vi "Standard Normal distribution.vi"() -> ()   [LabVIEW 2023]
uses:
  <vilib>/numeric/Random Number (Range) U64.vi
  <vilib>/numeric/Random Number (Range) DBL.vi
  <vilib>/numeric/sub_Random U32.vi
  <vilib>/gmath/NI_Gmath.lvlib
panel:
  in  "stop":bool
  out "xyGraph":cluster{"X":dbl, "Y":dbl}[](graph)=[{"X"=-6.09, "Y"=3.526399235495381e-09}, {"X"=-6.08, "Y"=3.747643729676039e-09}, {"X"=-6.07, "Y"=3.982370733890178e-09}, {"X"=-6.06, "Y"=4.231376288039894e-09}, {"X"=-6.05, "Y"=4.4955018310132455e-09}, {"X"=-6.04, "Y"=4.775636692282276e-09}, {"X"=-6.03, "Y"=5.072720714470481e-09}, {"X"=-6.02, "Y"=5.38774701344276e-09}, {"X"=-6.01, "Y"=5.7217648827798965e-09}, {"X"=-6.0, "Y"=6.075882849823286e-09}, {"X"=-5.99, "Y"=6.451271890811751e-09}, {"X"=-5.98, "Y"=6.8491688129857586e-09}, {"X"=-5.97, "Y"=7.270879811900108e-09}, {"X"=-5.96, "Y"=7.717784212570529e-09}, {"X"=-5.95, "Y"=8.191338403479174e-09}, {"X"=-5.94, "Y"=8.693079972880173e-09}, {"X"=-5.93, "Y"=9.22463205728272e-09}, {"X"=-5.92, "Y"=9.78770791244118e-09}, {"X"=-5.91, "Y"=1.0384115717656327e-08}, {"X"=-5.9, "Y"=1.1015763624682308e-08}, {"X"=-5.89, "Y"=1.168466506304987e-08}, {"X"=-5.88, "Y"=1.239294431415013e-08}, {"X"=-5.87, "Y"=1.3142842366982143e-08}, {"X"=-5.86, "Y"=1.3936723069047392e-08}, {"X"=-5.85, "Y"=1.4777079586480055e-08}, {"X"=-5.84, "Y"=1.5666541188132572e-08}, {"X"=-5.83, "Y"=1.6607880368992047e-08}, {"X"=-5.82, "Y"=1.7604020328985783e-08}, {"X"=-5.81, "Y"=1.865804282394618e-08}, {"X"=-5.8, "Y"=1.9773196406244675e-08}, {"X"=-5.79, "Y"=2.0952905073377047e-08}, {"X"=-5.78, "Y"=2.2200777343579013e-08}, {"X"=-5.77, "Y"=2.352061577839084e-08}, {"X"=-5.76, "Y"=2.4916426972950992e-08}, {"X"=-5.75, "Y"=2.6392432035705735e-08}, {"X"=-5.74, "Y"=2.795307758015465e-08}, {"X"=-5.73, "Y"=2.960304725223005e-08}, {"X"=-5.72, "Y"=3.134727381791979e-08}, {"X"=-5.71, "Y"=3.319095183679538e-08}, {"X"=-5.7, "Y"=3.513955094820434e-08}, {"X"=-5.69, "Y"=3.7198829798016034e-08}, {"X"=-5.68, "Y"=3.9374850634998504e-08}, {"X"=-5.67, "Y"=4.167399460712351e-08}, {"X"=-5.66, "Y"=4.410297778937308e-08}, {"X"=-5.65, "Y"=4.666886797594257e-08}, {"X"=-5.64, "Y"=4.937910227110449e-08}, {"X"=-5.63, "Y"=5.2241505514424374e-08}, {"X"=-5.62, "Y"=5.526430957749716e-08}, {"X"=-5.61, "Y"=5.84561735709005e-08}, {"X"=-5.6, "Y"=6.182620500165857e-08}, {"X"=-5.59, "Y"=6.538398192315145e-08}, {"X"=-5.58, "Y"=6.913957612112398e-08}, {"X"=-5.57, "Y"=7.310357738120935e-08}, {"X"=-5.56, "Y"=7.728711888522921e-08}, {"X"=-5.55, "Y"=8.17019037854322e-08}, {"X"=-5.54, "Y"=8.636023300780988e-08}, {"X"=-5.53, "Y"=9.127503433766477e-08}, {"X"=-5.52, "Y"=9.645989284273384e-08}, {"X"=-5.51, "Y"=1.0192908269135293e-07}, {"X"=-5.5, "Y"=1.0769760042543276e-07}, {"X"=-5.49, "Y"=1.1378119975034591e-07}, {"X"=-5.48, "Y"=1.201964279062823e-07}, {"X"=-5.47, "Y"=1.2696066368812932e-07}, {"X"=-5.46, "Y"=1.3409215718354753e-07}, {"X"=-5.45, "Y"=1.4161007130161178e-07}, {"X"=-5.44, "Y"=1.495345251671592e-07}, {"X"=-5.43, "Y"=1.5788663945889064e-07}, {"X"=-5.42, "Y"=1.6668858377222828e-07}, {"X"=-5.41, "Y"=1.7596362609104592e-07}, {"X"=-5.4, "Y"=1.8573618445552897e-07}, {"X"=-5.39, "Y"=1.9603188091675758e-07}, {"X"=-5.38, "Y"=2.0687759787196552e-07}, {"X"=-5.37, "Y"=2.1830153687797888e-07}, {"X"=-5.36, "Y"=2.3033328004392066e-07}, {"X"=-5.35, "Y"=2.4300385410805355e-07}, {"X"=-5.34, "Y"=2.5634579730745934e-07}, {"X"=-5.33, "Y"=2.7039322915329305e-07}, {"X"=-5.32, "Y"=2.851819232283976e-07}, {"X"=-5.31, "Y"=3.007493831283838e-07}, {"X"=-5.3, "Y"=3.171349216715976e-07}, {"X"=-5.29, "Y"=3.3437974350798003e-07}, {"X"=-5.28, "Y"=3.525270312614038e-07}, {"X"=-5.27, "Y"=3.7162203534495063e-07}, {"X"=-5.26, "Y"=3.9171216759348166e-07}, {"X"=-5.25, "Y"=4.1284709886299984e-07}, {"X"=-5.24, "Y"=4.350788607515109e-07}, {"X"=-5.23, "Y"=4.584619516015329e-07}, {"X"=-5.22, "Y"=4.830534469499683e-07}, {"X"=-5.21, "Y"=5.08913114596766e-07}, {"X"=-5.2, "Y"=5.361035344697615e-07}, {"X"=-5.19, "Y"=5.64690223469076e-07}, {"X"=-5.18, "Y"=5.947417654807764e-07}, {"X"=-5.17, "Y"=6.263299467558902e-07}, {"X"=-5.16, "Y"=6.595298968575217e-07}, {"X"=-5.15, "Y"=6.944202353855339e-07}, {"X"=-5.14, "Y"=7.310832246953503e-07}, {"X"=-5.13, "Y"=7.696049288345129e-07}, {"X"=-5.12, "Y"=8.100753789281346e-07}, {"X"=-5.11, "Y"=8.52588745251786e-07}, {"X"=-5.1, "Y"=8.972435162383337e-07}, {"X"=-5.09, "Y"=9.441426846730874e-07}, {"X"=-5.08, "Y"=9.93393941339912e-07}, {"X"=-5.07, "Y"=1.0451098763893177e-06}, {"X"=-5.06, "Y"=1.0994081887082052e-06}, {"X"=-5.05, "Y"=1.1564119035797834e-06}, {"X"=-5.04, "Y"=1.216249598931318e-06}, {"X"=-5.03, "Y"=1.2790556404765742e-06}, {"X"=-5.02, "Y"=1.3449704260694445e-06}, {"X"=-5.01, "Y"=1.4141406395950037e-06}, {"X"=-5.0, "Y"=1.4867195147342979e-06}, {"X"=-4.99, "Y"=1.5628671089492902e-06}, {"X"=-4.98, "Y"=1.6427505880450713e-06}, {"X"=-4.97, "Y"=1.7265445216770736e-06}, {"X"=-4.96, "Y"=1.8144311901820306e-06}, {"X"=-4.95, "Y"=1.906600903122811e-06}, {"X"=-4.94, "Y"=2.0032523299484894e-06}, {"X"=-4.93, "Y"=2.10459284318313e-06}, {"X"=-4.92, "Y"=2.2108388745684212e-06}, {"X"=-4.91, "Y"=2.322216284597997e-06}, {"X"=-4.9, "Y"=2.438960745893352e-06}, {"X"=-4.89, "Y"=2.5613181408845447e-06}, {"X"=-4.88, "Y"=2.6895449742715237e-06}, {"X"=-4.87, "Y"=2.823908800755821e-06}, {"X"=-4.86, "Y"=2.964688668545273e-06}, {"X"=-4.85, "Y"=3.112175579148945e-06}, {"X"=-4.84, "Y"=3.266672963993275e-06}, {"X"=-4.83, "Y"=3.428497178405039e-06}, {"X"=-4.82, "Y"=3.5979780135212474e-06}, {"X"=-4.81, "Y"=3.775459226701349e-06}, {"X"=-4.8, "Y"=3.961299091032075e-06}, {"X"=-4.79, "Y"=4.155870964531201e-06}, {"X"=-4.78, "Y"=4.359563879671637e-06}, {"X"=-4.77, "Y"=4.5727831538641446e-06}, {"X"=-4.76, "Y"=4.795951021552522e-06}, {"X"=-4.75, "Y"=5.029507288592446e-06}, {"X"=-4.74, "Y"=5.273910009601304e-06}, {"X"=-4.73, "Y"=5.529636188984052e-06}, {"X"=-4.72, "Y"=5.797182506357288e-06}, {"X"=-4.71, "Y"=6.077066067111116e-06}, {"X"=-4.7, "Y"=6.36982517886709e-06}, {"X"=-4.69, "Y"=6.676020154607462e-06}, {"X"=-4.68, "Y"=6.996234143270405e-06}, {"X"=-4.67, "Y"=7.331073988623946e-06}, {"X"=-4.66, "Y"=7.681171117250455e-06}, {"X"=-4.65, "Y"=8.047182456492295e-06}, {"X"=-4.64, "Y"=8.429791383228772e-06}, {"X"=-4.63, "Y"=8.829708704374098e-06}, {"X"=-4.62, "Y"=9.247673670005617e-06}, {"X"=-4.61, "Y"=9.684455020051437e-06}, {"X"=-4.6, "Y"=1.014085206548676e-05}, {"X"=-4.59, "Y"=1.0617695805008393e-05}, {"X"=-4.58, "Y"=1.111585007817779e-05}, {"X"=-4.57, "Y"=1.1636212756042669e-05}, {"X"=-4.56, "Y"=1.21797169702687e-05}, {"X"=-4.55, "Y"=1.2747332381833467e-05}, {"X"=-4.54, "Y"=1.334006649035584e-05}, {"X"=-4.53, "Y"=1.3958965985154772e-05}, {"X"=-4.52, "Y"=1.4605118139152942e-05}, {"X"=-4.51, "Y"=1.527965224676162e-05}, {"X"=-4.5, "Y"=1.5983741106905478e-05}, {"X"=-4.49, "Y"=1.671860255236507e-05}, {"X"=-4.48, "Y"=1.748550102663914e-05}, {"X"=-4.47, "Y"=1.828574920954738e-05}, {"X"=-4.46, "Y"=1.9120709692817737e-05}, {"X"=-4.45, "Y"=1.999179670692279e-05}, {"X"=-4.44, "Y"=2.0900477900450407e-05}, {"X"=-4.43, "Y"=2.184827617331647e-05}, {"X"=-4.42, "Y"=2.283677156514692e-05}, {"X"=-4.41, "Y"=2.38676032001796e-05}, {"X"=-4.4, "Y"=2.4942471290053535e-05}, {"X"=-4.39, "Y"=2.6063139195878346e-05}, {"X"=-4.38, "Y"=2.723143555099261e-05}, {"X"=-4.37, "Y"=2.8449256445844308e-05}, {"X"=-4.36, "Y"=2.97185676764422e-05}, {"X"=-4.35, "Y"=3.1041407057850266e-05}, {"X"=-4.34, "Y"=3.241988680421378e-05}, {"X"=-4.33, "Y"=3.385619597682789e-05}, {"X"=-4.32, "Y"=3.5352603001773097e-05}, {"X"=-4.31, "Y"=3.69114582586662e-05}, {"X"=-4.3, "Y"=3.853519674208713e-05}, {"X"=-4.29, "Y"=4.022634079726497e-05}, {"X"=-4.28, "Y"=4.198750293161732e-05}, {"X"=-4.27, "Y"=4.382138870375812e-05}, {"X"=-4.26, "Y"=4.5730799691601314e-05}, {"X"=-4.25, "Y"=4.771863654120495e-05}, {"X"=-4.24, "Y"=4.978790209801209e-05}, {"X"=-4.23, "Y"=5.1941704622159776e-05}, {"X"=-4.22, "Y"=5.4183261089540144e-05}, {"X"=-4.21, "Y"=5.651590058030741e-05}, {"X"=-4.2, "Y"=5.8943067756539855e-05}, {"X"=-4.19, "Y"=6.146832643076922e-05}, {"X"=-4.18, "Y"=6.40953632271061e-05}, {"X"=-4.17, "Y"=6.682799133669061e-05}, {"X"=-4.16, "Y"=6.967015436921434e-05}, {"X"=-4.15, "Y"=7.262593030225234e-05}, {"X"=-4.14, "Y"=7.569953553016121e-05}, {"X"=-4.13, "Y"=7.889532901429309e-05}, {"X"=-4.12, "Y"=8.2217816536286e-05}, {"X"=-4.11, "Y"=8.567165505618186e-05}, {"X"=-4.1, "Y"=8.926165717713293e-05}, {"X"=-4.09, "Y"=9.299279571844591e-05}, {"X"=-4.08, "Y"=9.687020839871927e-05}, {"X"=-4.07, "Y"=0.00010089920263081443}, {"X"=-4.06, "Y"=0.00010508526043040049}, {"X"=-4.05, "Y"=0.00010943404343980055}, {"X"=-4.04, "Y"=0.00011395139806886461}, {"X"=-4.03, "Y"=0.00011864336075456578}, {"X"=-4.02, "Y"=0.00012351616334102368}, {"X"=-4.01, "Y"=0.00012857623858162108}, {"X"=-4.0, "Y"=0.00013383022576488537}, {"X"=-3.99, "Y"=0.00013928497646575994}, {"X"=-3.98, "Y"=0.00014494756042389106}, {"X"=-3.97, "Y"=0.0001508252715505178}, {"X"=-3.96, "Y"=0.00015692563406553226}, {"X"=-3.95, "Y"=0.00016325640876624202}, {"X"=-3.94, "Y"=0.00016982559942934359}, {"X"=-3.93, "Y"=0.00017664145934757092}, {"X"=-3.92, "Y"=0.0001837124980024571}, {"X"=-3.91, "Y"=0.00019104748787459762}, {"X"=-3.9, "Y"=0.00019865547139277272}, {"X"=-3.89, "Y"=0.00020654576802322548}, {"X"=-3.88, "Y"=0.00021472798150036704}, {"X"=-3.87, "Y"=0.0002232120072001021}, {"X"=-3.86, "Y"=0.00023200803965694238}, {"X"=-3.85, "Y"=0.00024112658022599324}, {"X"=-3.84, "Y"=0.00025057844489086075}, {"X"=-3.83, "Y"=0.00026037477221844247}, {"X"=-3.82, "Y"=0.000270527031461521}, {"X"=-3.81, "Y"=0.0002810470308099863}, {"X"=-3.8, "Y"=0.00029194692579146027}, {"X"=-3.79, "Y"=0.0003032392278220042}, {"X"=-3.78, "Y"=0.0003149368129075219}, {"X"=-3.77, "Y"=0.00032705293049637503}, {"X"=-3.76, "Y"=0.0003396012124836548}, {"X"=-3.75, "Y"=0.00035259568236744546}, {"X"=-3.74, "Y"=0.000366050764557335}, {"X"=-3.73, "Y"=0.00037998129383532146}, {"X"=-3.72, "Y"=0.0003944025249691562}, {"X"=-3.71, "Y"=0.0004093301424780789}, {"X"=-3.7, "Y"=0.00042478027055075143}, {"X"=-3.69, "Y"=0.0004407694831151325}, {"X"=-3.68, "Y"=0.00045731481405985675}, {"X"=-3.67, "Y"=0.00047443376760662064}, {"X"=-3.66, "Y"=0.0004921443288328931}, {"X"=-3.65, "Y"=0.0005104649743441856}, {"X"=-3.64, "Y"=0.0005294146830949348}, {"X"=-3.63, "Y"=0.0005490129473569587}, {"X"=-3.62, "Y"=0.0005692797838342526}, {"X"=-3.61, "Y"=0.0005902357449227856}, {"X"=-3.6, "Y"=0.0006119019301137719}, {"X"=-3.59, "Y"=0.0006342999975387576}, {"X"=-3.58, "Y"=0.0006574521756546766}, {"X"=-3.57, "Y"=0.0006813812750668921}, {"X"=-3.56, "Y"=0.0007061107004880362}, {"X"=-3.55, "Y"=0.0007316644628303109}, {"X"=-3.54, "Y"=0.0007580671914287103}, {"X"=-3.53, "Y"=0.00078534414639247}, {"X"=-3.52, "Y"=0.0008135212310818085}, {"X"=-3.51, "Y"=0.0008426250047069028}, {"X"=-3.5, "Y"=0.0008726826950457602}, {"X"=-3.49, "Y"=0.0009037222112775245}, {"X"=-3.48, "Y"=0.0009357721569274798}, {"X"=-3.47, "Y"=0.0009688618429198459}, {"X"=-3.46, "Y"=0.0010030213007342376}, {"X"=-3.45, "Y"=0.0010382812956614103}, {"X"=-3.44, "Y"=0.0010746733401537356}, {"X"=-3.43, "Y"=0.0011122297072655649}, {"X"=-3.42, "Y"=0.0011509834441784845}, {"X"=-3.41, "Y"=0.0011909683858061168}, {"X"=-3.4, "Y"=0.00123221916847302}, {"X"=-3.39, "Y"=0.001274771243661833}, {"X"=-3.38, "Y"=0.0013186608918227423}, {"X"=-3.37, "Y"=0.0013639252362389036}, {"X"=-3.36, "Y"=0.001410602256941385}, {"X"=-3.35, "Y"=0.0014587308046667459}, {"X"=-3.34, "Y"=0.0015083506148503075}, {"X"=-3.33, "Y"=0.0015595023216476915}, {"X"=-3.32, "Y"=0.0016122274719771244}, {"X"=-3.31, "Y"=0.0016665685395745797}, {"X"=-3.3, "Y"=0.0017225689390536812}, {"X"=-3.29, "Y"=0.0017802730399618788}, {"X"=-3.28, "Y"=0.0018397261808242812}, {"X"=-3.27, "Y"=0.0019009746831660803}, {"X"=-3.26, "Y"=0.001964065865504376}, {"X"=-3.25, "Y"=0.002029048057299768}, {"X"=-3.24, "Y"=0.002095970612857942}, {"X"=-3.23, "Y"=0.0021648839251710624}, {"X"=-3.22, "Y"=0.0022358394396885385}, {"X"=-3.21, "Y"=0.0023088896680064958}, {"X"=-3.2, "Y"=0.0023840882014648404}, {"X"=-3.19, "Y"=0.0024614897246407006}, {"X"=-3.18, "Y"=0.002541150028726522}, {"X"=-3.17, "Y"=0.0026231260247810244}, {"X"=-3.16, "Y"=0.0027074757568407003}, {"X"=-3.15, "Y"=0.002794258414879447}, {"X"=-3.14, "Y"=0.002883534347603439}, {"X"=-3.13, "Y"=0.002975365075068254}, {"X"=-3.12, "Y"=0.0030698133011047403}, {"X"=-3.11, "Y"=0.0031669429255400815}, {"X"=-3.1, "Y"=0.0032668190561999186}, {"X"=-3.09, "Y"=0.0033695080206774812}, {"X"=-3.08, "Y"=0.003475077377854938}, {"X"=-3.07, "Y"=0.0035835959291623614}, {"X"=-3.06, "Y"=0.003695133729559035}, {"X"=-3.05, "Y"=0.0038097620982218104}, {"X"=-3.04, "Y"=0.003927553628924779}, {"X"=-3.03, "Y"=0.00404858220009443}, {"X"=-3.02, "Y"=0.004172922984523962}, {"X"=-3.01, "Y"=0.00430065245873045}, {"X"=-3.0, "Y"=0.0044318484119380075}, {"X"=-2.99, "Y"=0.004566589954670145}, {"X"=-2.98, "Y"=0.004704957526933979}, {"X"=-2.97, "Y"=0.004847032905978945}, {"X"=-2.96, "Y"=0.004992899213612376}, {"X"=-2.95, "Y"=0.005142640923053939}, {"X"=-2.94, "Y"=0.00529634386531102}, {"X"=-2.93, "Y"=0.005454095235056545}, {"X"=-2.92, "Y"=0.005615983595990969}, {"X"=-2.91, "Y"=0.005782098885669473}, {"X"=-2.9, "Y"=0.005952532419775854}, {"X"=-2.89, "Y"=0.006127376895823688}, {"X"=-2.88, "Y"=0.0063067263962659275}, {"X"=-2.87, "Y"=0.006490676390993364}, {"X"=-2.86, "Y"=0.00667932373920262}, {"X"=-2.85, "Y"=0.006872766690613971}, {"X"=-2.84, "Y"=0.007071104886019449}, {"X"=-2.83, "Y"=0.007274439357141218}, {"X"=-2.82, "Y"=0.007482872525780564}, {"X"=-2.81, "Y"=0.007696508202237322}, {"X"=-2.8, "Y"=0.007915451582979969}, {"X"=-2.79, "Y"=0.008139809247546021}, {"X"=-2.78, "Y"=0.008369689154653033}, {"X"=-2.77, "Y"=0.008605200637499673}, {"X"=-2.76, "Y"=0.008846454398237232}, {"X"=-2.75, "Y"=0.009093562501591053}, {"X"=-2.74, "Y"=0.009346638367612283}, {"X"=-2.73, "Y"=0.009605796763539587}, {"X"=-2.72, "Y"=0.009871153794751132}, {"X"=-2.71, "Y"=0.010142826894787078}, {"X"=-2.7, "Y"=0.010420934814422592}, {"X"=-2.69, "Y"=0.010705597609772188}, {"X"=-2.68, "Y"=0.010996936629405572}, {"X"=-2.67, "Y"=0.011295074500456135}, {"X"=-2.66, "Y"=0.011600135113702562}, {"X"=-2.65, "Y"=0.01191224360760518}, {"X"=-2.64, "Y"=0.012231526351277971}, {"X"=-2.63, "Y"=0.012558110926378211}, {"X"=-2.62, "Y"=0.012892126107895304}, {"X"=-2.61, "Y"=0.013233701843821374}, {"X"=-2.6, "Y"=0.013582969233685615}, {"X"=-2.59, "Y"=0.013940060505935825}, {"X"=-2.58, "Y"=0.014305108994149692}, {"X"=-2.57, "Y"=0.014678249112060044}, {"X"=-2.56, "Y"=0.01505961632737745}, {"X"=-2.55, "Y"=0.015449347134395174}, {"X"=-2.54, "Y"=0.015847579025360818}, {"X"=-2.53, "Y"=0.016254450460600506}, {"X"=-2.52, "Y"=0.016670100837381057}, {"X"=-2.51, "Y"=0.017094670457496956}, {"X"=-2.5, "Y"=0.01752830049356854}, {"X"=-2.49, "Y"=0.017971132954039633}, {"X"=-2.48, "Y"=0.01842331064686205}, {"X"=-2.47, "Y"=0.018884977141856163}, {"X"=-2.46, "Y"=0.019356276731736965}, {"X"=-2.45, "Y"=0.019837354391795313}, {"X"=-2.44, "Y"=0.02032835573822584}, {"X"=-2.43, "Y"=0.020829426985092186}, {"X"=-2.42, "Y"=0.021340714899922786}, {"X"=-2.41, "Y"=0.021862366757929387}, {"X"=-2.4, "Y"=0.0223945302948429}, {"X"=-2.39, "Y"=0.022937353658360693}, {"X"=-2.38, "Y"=0.023490985358201367}, {"X"=-2.37, "Y"=0.02405557421476297}, {"X"=-2.36, "Y"=0.024631269306382507}, {"X"=-2.35, "Y"=0.025218219915194382}, {"X"=-2.34, "Y"=0.02581657547158769}, {"X"=-2.33, "Y"=0.026426485497261724}, {"X"=-2.32, "Y"=0.027048099546881785}, {"X"=-2.31, "Y"=0.027681567148336573}, {"X"=-2.3, "Y"=0.02832703774160119}, {"X"=-2.29, "Y"=0.028984660616209416}, {"X"=-2.28, "Y"=0.029654584847341278}, {"X"=-2.27, "Y"=0.03033695923053164}, {"X"=-2.26, "Y"=0.031031932215008273}, {"X"=-2.25, "Y"=0.03173965183566742}, {"X"=-2.24, "Y"=0.032460265643697445}, {"X"=-2.23, "Y"=0.03319392063586112}, {"X"=-2.22, "Y"=0.033940763182449186}, {"X"=-2.21, "Y"=0.03470093895391882}, {"X"=-2.2, "Y"=0.035474592846231424}, {"X"=-2.19, "Y"=0.03626186890490622}, {"X"=-2.18, "Y"=0.037062910247806474}, {"X"=-2.17, "Y"=0.03787785898667748}, {"X"=-2.16, "Y"=0.03870685614745561}, {"X"=-2.15, "Y"=0.03955004158937022}, {"X"=-2.14, "Y"=0.04040755392286031}, {"X"=-2.13, "Y"=0.041279530426330424}, {"X"=-2.12, "Y"=0.04216610696177031}, {"X"=-2.11, "Y"=0.04306741788926574}, {"X"=-2.1, "Y"=0.0439835959804272}, {"X"=-2.09, "Y"=0.0449147723307671}, {"X"=-2.08, "Y"=0.045861076271054894}, {"X"=-2.07, "Y"=0.04682263527768316}, {"X"=-2.06, "Y"=0.047799574882077034}, {"X"=-2.05, "Y"=0.04879201857918277}, {"X"=-2.04, "Y"=0.049800087735070775}, {"X"=-2.03, "Y"=0.05082390149369121}, {"X"=-2.02, "Y"=0.051863576682820565}, {"X"=-2.01, "Y"=0.05291922771924032}, {"X"=-2.0, "Y"=0.05399096651318806}, {"X"=-1.99, "Y"=0.05507890237212577}, {"X"=-1.98, "Y"=0.05618314190386805}, {"X"=-1.97, "Y"=0.05730378891911713}, {"X"=-1.96, "Y"=0.058440944333451476}, {"X"=-1.95, "Y"=0.059594706068816075}, {"X"=-1.94, "Y"=0.06076516895456478}, {"X"=-1.93, "Y"=0.061952424628105164}, {"X"=-1.92, "Y"=0.06315656143519865}, {"X"=-1.91, "Y"=0.06437766432996936}, {"X"=-1.9, "Y"=0.0656158147746766}, {"X"=-1.89, "Y"=0.06687109063930716}, {"X"=-1.88, "Y"=0.06814356610104459}, {"X"=-1.87, "Y"=0.06943331154367419}, {"X"=-1.86, "Y"=0.07074039345698338}, {"X"=-1.85, "Y"=0.072064874336218}, {"X"=-1.84, "Y"=0.07340681258165689}, {"X"=-1.83, "Y"=0.0747662623983676}, {"X"=-1.82, "Y"=0.07614327369620731}, {"X"=-1.81, "Y"=0.07753789199013399}, {"X"=-1.8, "Y"=0.07895015830089415}, {"X"=-1.79, "Y"=0.08038010905615417}, {"X"=-1.78, "Y"=0.08182777599214282}, {"X"=-1.77, "Y"=0.08329318605587446}, {"X"=-1.76, "Y"=0.08477636130802224}, {"X"=-1.75, "Y"=0.08627731882651153}, {"X"=-1.74, "Y"=0.08779607061090564}, {"X"=-1.73, "Y"=0.089332623487655}, {"X"=-1.72, "Y"=0.09088697901628288}, {"X"=-1.71, "Y"=0.09245913339658068}, {"X"=-1.7, "Y"=0.09404907737688695}, {"X"=-1.69, "Y"=0.09565679616352402}, {"X"=-1.68, "Y"=0.09728226933146752}, {"X"=-1.67, "Y"=0.09892547073632373}, {"X"=-1.66, "Y"=0.10058636842769057}, {"X"=-1.65, "Y"=0.10226492456397804}, {"X"=-1.64, "Y"=0.10396109532876424}, {"X"=-1.63, "Y"=0.10567483084876363}, {"X"=-1.62, "Y"=0.1074060751134838}, {"X"=-1.61, "Y"=0.10915476589664735}, {"X"=-1.6, "Y"=0.11092083467945554}, {"X"=-1.59, "Y"=0.11270420657577056}, {"X"=-1.58, "Y"=0.11450480025929236}, {"X"=-1.57, "Y"=0.1163225278928071}, {"X"=-1.56, "Y"=0.11815729505958228}, {"X"=-1.55, "Y"=0.12000900069698558}, {"X"=-1.54, "Y"=0.12187753703240178}, {"X"=-1.53, "Y"=0.12376278952152314}, {"X"=-1.52, "Y"=0.12566463678908815}, {"X"=-1.51, "Y"=0.12758295057214186}, {"X"=-1.5, "Y"=0.12951759566589174}, {"X"=-1.49, "Y"=0.13146842987223106}, {"X"=-1.48, "Y"=0.13343530395100234}, {"X"=-1.47, "Y"=0.1354180615740713}, {"X"=-1.46, "Y"=0.13741653928228179}, {"X"=-1.45, "Y"=0.13943056644536028}, {"X"=-1.44, "Y"=0.1414599652248388}, {"X"=-1.43, "Y"=0.14350455054006242}, {"X"=-1.42, "Y"=0.1455641300373476}, {"X"=-1.41, "Y"=0.14763850406235574}, {"X"=-1.4, "Y"=0.14972746563574488}, {"X"=-1.39, "Y"=0.1518308004321617}, {"X"=-1.38, "Y"=0.15394828676263372}, {"X"=-1.37, "Y"=0.15607969556042084}, {"X"=-1.36, "Y"=0.15822479037038303}, {"X"=-1.35, "Y"=0.1603833273419196}, {"X"=-1.34, "Y"=0.16255505522553412}, {"X"=-1.33, "Y"=0.1647397153730768}, {"X"=-1.32, "Y"=0.1669370417417138}, {"X"=-1.31, "Y"=0.1691467609016724}, {"X"=-1.3, "Y"=0.17136859204780736}, {"X"=-1.29, "Y"=0.173602247015033}, {"X"=-1.28, "Y"=0.17584743029766237}, {"X"=-1.27, "Y"=0.1781038390726936}, {"X"=-1.26, "Y"=0.18037116322708033}, {"X"=-1.25, "Y"=0.18264908538902191}, {"X"=-1.24, "Y"=0.1849372809633053}, {"X"=-1.23, "Y"=0.18723541817072956}, {"X"=-1.22, "Y"=0.18954315809164027}, {"X"=-1.21, "Y"=0.1918601547135994}, {"X"=-1.2, "Y"=0.19418605498321298}, {"X"=-1.19, "Y"=0.19652049886213654}, {"X"=-1.18, "Y"=0.1988631193872759}, {"X"=-1.17, "Y"=0.2012135427351974}, {"X"=-1.16, "Y"=0.20357138829075944}, {"X"=-1.15, "Y"=0.20593626871997478}, {"X"=-1.14, "Y"=0.20830779004710837}, {"X"=-1.13, "Y"=0.21068555173601533}, {"X"=-1.12, "Y"=0.21306914677571784}, {"X"=-1.11, "Y"=0.2154581617702197}, {"X"=-1.1, "Y"=0.21785217703255055}, {"X"=-1.09, "Y"=0.22025076668303326}, {"X"=-1.08, "Y"=0.22265349875176116}, {"X"=-1.07, "Y"=0.22505993528526969}, {"X"=-1.06, "Y"=0.2274696324573859}, {"X"=-1.05, "Y"=0.22988214068423302}, {"X"=-1.04, "Y"=0.2322970047433662}, {"X"=-1.03, "Y"=0.23471376389701185}, {"X"=-1.02, "Y"=0.23713195201937962}, {"X"=-1.01, "Y"=0.23955109772801336}, {"X"=-1.0, "Y"=0.24197072451914337}, {"X"=-0.99, "Y"=0.2443903509069996}, {"X"=-0.98, "Y"=0.24680949056704274}, {"X"=-0.97, "Y"=0.24922765248306594}, {"X"=-0.96, "Y"=0.2516443410981171}, {"X"=-0.95, "Y"=0.254059056469189}, {"X"=-0.94, "Y"=0.25647129442562033}, {"X"=-0.93, "Y"=0.25888054673114885}, {"X"=-0.92, "Y"=0.26128630124955315}, {"X"=-0.91, "Y"=0.2636880421138182}, {"X"=-0.9, "Y"=0.2660852498987548}, {"X"=-0.89, "Y"=0.2684774017970024}, {"X"=-0.88, "Y"=0.27086397179833804}, {"X"=-0.87, "Y"=0.2732444308722162}, {"X"=-0.86, "Y"=0.27561824715345673}, {"X"=-0.85, "Y"=0.2779848861309965}, {"X"=-0.84, "Y"=0.2803438108396206}, {"X"=-0.83, "Y"=0.28269448205458025}, {"X"=-0.82, "Y"=0.28503635848900727}, {"X"=-0.81, "Y"=0.2873688969940283}, {"X"=-0.8, "Y"=0.28969155276148273}, {"X"=-0.79, "Y"=0.2920037795291414}, {"X"=-0.78, "Y"=0.2943050297883251}, {"X"=-0.77, "Y"=0.2965947549938157}, {"X"=-0.76, "Y"=0.29887240577595275}, {"X"=-0.75, "Y"=0.30113743215480443}, {"X"=-0.74, "Y"=0.30338928375630014}, {"X"=-0.73, "Y"=0.30562741003020993}, {"X"=-0.72, "Y"=0.30785126046985295}, {"X"=-0.71, "Y"=0.31006028483341613}, {"X"=-0.7, "Y"=0.31225393336676127}, {"X"=-0.69, "Y"=0.31443165702759734}, {"X"=-0.68, "Y"=0.31659290771089277}, {"X"=-0.67, "Y"=0.3187371384754015}, {"X"=-0.66, "Y"=0.3208638037711725}, {"X"=-0.65, "Y"=0.3229723596679143}, {"X"=-0.64, "Y"=0.3250622640840822}, {"X"=-0.63, "Y"=0.3271329770165545}, {"X"=-0.62, "Y"=0.3291839607707648}, {"X"=-0.61, "Y"=0.33121468019115297}, {"X"=-0.6, "Y"=0.33322460289179967}, {"X"=-0.59, "Y"=0.33521319948710615}, {"X"=-0.58, "Y"=0.3371799438223806}, {"X"=-0.57, "Y"=0.33912431320419223}, {"X"=-0.56, "Y"=0.34104578863035256}, {"X"=-0.55, "Y"=0.3429438550193839}, {"X"=-0.54, "Y"=0.3448180014393334}, {"X"=-0.53, "Y"=0.34666772133579166}, {"X"=-0.52, "Y"=0.3484925127589745}, {"X"=-0.51, "Y"=0.3502918785897258}, {"X"=-0.5, "Y"=0.3520653267642995}, {"X"=-0.49, "Y"=0.3538123704977797}, {"X"=-0.48, "Y"=0.3555325285059971}, {"X"=-0.47, "Y"=0.35722532522580086}, {"X"=-0.46, "Y"=0.35889029103354464}, {"X"=-0.45, "Y"=0.36052696246164795}, {"X"=-0.44, "Y"=0.3621348824130922}, {"X"=-0.43, "Y"=0.3637136003737134}, {"X"=-0.42, "Y"=0.3652626726221539}, {"X"=-0.41, "Y"=0.3667816624373361}, {"X"=-0.4, "Y"=0.36827014030332333}, {"X"=-0.39, "Y"=0.36972768411143236}, {"X"=-0.38, "Y"=0.37115387935946603}, {"X"=-0.37, "Y"=0.3725483193479334}, {"X"=-0.36, "Y"=0.3739106053731284}, {"X"=-0.35, "Y"=0.3752403469169379}, {"X"=-0.34, "Y"=0.376537161833254}, {"X"=-0.33, "Y"=0.37780067653086463}, {"X"=-0.32, "Y"=0.3790305261527017}, {"X"=-0.31, "Y"=0.38022635475132494}, {"X"=-0.3, "Y"=0.38138781546052414}, {"X"=-0.29, "Y"=0.38251457066292405}, {"X"=-0.28, "Y"=0.3836062921534786}, {"X"=-0.27, "Y"=0.3846626612987428}, {"X"=-0.26, "Y"=0.3856833691918161}, {"X"=-0.25, "Y"=0.3866681168028493}, {"X"=-0.24, "Y"=0.38761661512501416}, {"X"=-0.23, "Y"=0.3885285853158359}, {"X"=-0.22, "Y"=0.38940375883379047}, {"X"=-0.21, "Y"=0.39024187757007434}, {"X"=-0.2, "Y"=0.3910426939754559}, {"X"=-0.19, "Y"=0.3918059711821211}, {"X"=-0.18, "Y"=0.3925314831204289}, {"X"=-0.17, "Y"=0.3932190146304972}, {"X"=-0.16, "Y"=0.3938683615685408}, {"X"=-0.15, "Y"=0.39447933090788895}, {"X"=-0.14, "Y"=0.39505174083461125}, {"X"=-0.13, "Y"=0.3955854208376874}, {"X"=-0.12, "Y"=0.3960802117936561}, {"X"=-0.11, "Y"=0.3965359660456858}, {"X"=-0.1, "Y"=0.3969525474770118}, {"X"=-0.09, "Y"=0.39732983157868834}, {"X"=-0.08, "Y"=0.3976677055116089}, {"X"=-0.07, "Y"=0.39796606816275104}, {"X"=-0.06, "Y"=0.39822483019560695}, {"X"=-0.05, "Y"=0.39844391409476404}, {"X"=-0.04, "Y"=0.39862325420460504}, {"X"=-0.03, "Y"=0.39876279676209975}, {"X"=-0.02, "Y"=0.3988624999236661}, {"X"=-0.01, "Y"=0.39892233378608216}, {"X"=0.0, "Y"=0.3989422804014327}, {"X"=-0.0, "Y"=0.3989422804014327}, {"X"=0.01, "Y"=0.39892233378608216}, {"X"=0.02, "Y"=0.3988624999236661}, {"X"=0.03, "Y"=0.39876279676209975}, {"X"=0.04, "Y"=0.39862325420460504}, {"X"=0.05, "Y"=0.39844391409476404}, {"X"=0.06, "Y"=0.39822483019560695}, {"X"=0.07, "Y"=0.39796606816275104}, {"X"=0.08, "Y"=0.3976677055116089}, {"X"=0.09, "Y"=0.39732983157868834}, {"X"=0.1, "Y"=0.3969525474770118}, {"X"=0.11, "Y"=0.3965359660456858}, {"X"=0.12, "Y"=0.3960802117936561}, {"X"=0.13, "Y"=0.3955854208376874}, {"X"=0.14, "Y"=0.39505174083461125}, {"X"=0.15, "Y"=0.39447933090788895}, {"X"=0.16, "Y"=0.3938683615685408}, {"X"=0.17, "Y"=0.3932190146304972}, {"X"=0.18, "Y"=0.3925314831204289}, {"X"=0.19, "Y"=0.3918059711821211}, {"X"=0.2, "Y"=0.3910426939754559}, {"X"=0.21, "Y"=0.39024187757007434}, {"X"=0.22, "Y"=0.38940375883379047}, {"X"=0.23, "Y"=0.3885285853158359}, {"X"=0.24, "Y"=0.38761661512501416}, {"X"=0.25, "Y"=0.3866681168028493}, {"X"=0.26, "Y"=0.3856833691918161}, {"X"=0.27, "Y"=0.3846626612987428}, {"X"=0.28, "Y"=0.3836062921534786}, {"X"=0.29, "Y"=0.38251457066292405}, {"X"=0.3, "Y"=0.38138781546052414}, {"X"=0.31, "Y"=0.38022635475132494}, {"X"=0.32, "Y"=0.3790305261527017}, {"X"=0.33, "Y"=0.37780067653086463}, {"X"=0.34, "Y"=0.376537161833254}, {"X"=0.35, "Y"=0.3752403469169379}, {"X"=0.36, "Y"=0.3739106053731284}, {"X"=0.37, "Y"=0.3725483193479334}, {"X"=0.38, "Y"=0.37115387935946603}, {"X"=0.39, "Y"=0.36972768411143236}, {"X"=0.4, "Y"=0.36827014030332333}, {"X"=0.41, "Y"=0.3667816624373361}, {"X"=0.42, "Y"=0.3652626726221539}, {"X"=0.43, "Y"=0.3637136003737134}, {"X"=0.44, "Y"=0.3621348824130922}, {"X"=0.45, "Y"=0.36052696246164795}, {"X"=0.46, "Y"=0.35889029103354464}, {"X"=0.47, "Y"=0.35722532522580086}, {"X"=0.48, "Y"=0.3555325285059971}, {"X"=0.49, "Y"=0.3538123704977797}, {"X"=0.5, "Y"=0.3520653267642995}, {"X"=0.51, "Y"=0.3502918785897258}, {"X"=0.52, "Y"=0.3484925127589745}, {"X"=0.53, "Y"=0.34666772133579166}, {"X"=0.54, "Y"=0.3448180014393334}, {"X"=0.55, "Y"=0.3429438550193839}, {"X"=0.56, "Y"=0.34104578863035256}, {"X"=0.57, "Y"=0.33912431320419223}, {"X"=0.58, "Y"=0.3371799438223806}, {"X"=0.59, "Y"=0.33521319948710615}, {"X"=0.6, "Y"=0.33322460289179967}, {"X"=0.61, "Y"=0.33121468019115297}, {"X"=0.62, "Y"=0.3291839607707648}, {"X"=0.63, "Y"=0.3271329770165545}, {"X"=0.64, "Y"=0.3250622640840822}, {"X"=0.65, "Y"=0.3229723596679143}, {"X"=0.66, "Y"=0.3208638037711725}, {"X"=0.67, "Y"=0.3187371384754015}, {"X"=0.68, "Y"=0.31659290771089277}, {"X"=0.69, "Y"=0.31443165702759734}, {"X"=0.7, "Y"=0.31225393336676127}, {"X"=0.71, "Y"=0.31006028483341613}, {"X"=0.72, "Y"=0.30785126046985295}, {"X"=0.73, "Y"=0.30562741003020993}, {"X"=0.74, "Y"=0.30338928375630014}, {"X"=0.75, "Y"=0.30113743215480443}, {"X"=0.76, "Y"=0.29887240577595275}, {"X"=0.77, "Y"=0.2965947549938157}, {"X"=0.78, "Y"=0.2943050297883251}, {"X"=0.79, "Y"=0.2920037795291414}, {"X"=0.8, "Y"=0.28969155276148273}, {"X"=0.81, "Y"=0.2873688969940283}, {"X"=0.82, "Y"=0.28503635848900727}, {"X"=0.83, "Y"=0.28269448205458025}, {"X"=0.84, "Y"=0.2803438108396206}, {"X"=0.85, "Y"=0.2779848861309965}, {"X"=0.86, "Y"=0.27561824715345673}, {"X"=0.87, "Y"=0.2732444308722162}, {"X"=0.88, "Y"=0.27086397179833804}, {"X"=0.89, "Y"=0.2684774017970024}, {"X"=0.9, "Y"=0.2660852498987548}, {"X"=0.91, "Y"=0.2636880421138182}, {"X"=0.92, "Y"=0.26128630124955315}, {"X"=0.93, "Y"=0.25888054673114885}, {"X"=0.94, "Y"=0.25647129442562033}, {"X"=0.95, "Y"=0.254059056469189}, {"X"=0.96, "Y"=0.2516443410981171}, {"X"=0.97, "Y"=0.24922765248306594}, {"X"=0.98, "Y"=0.24680949056704274}, {"X"=0.99, "Y"=0.2443903509069996}, {"X"=1.0, "Y"=0.24197072451914337}, {"X"=1.01, "Y"=0.23955109772801336}, {"X"=1.02, "Y"=0.23713195201937962}, {"X"=1.03, "Y"=0.23471376389701185}, {"X"=1.04, "Y"=0.2322970047433662}, {"X"=1.05, "Y"=0.22988214068423302}, {"X"=1.06, "Y"=0.2274696324573859}, {"X"=1.07, "Y"=0.22505993528526969}, {"X"=1.08, "Y"=0.22265349875176116}, {"X"=1.09, "Y"=0.22025076668303326}, {"X"=1.1, "Y"=0.21785217703255055}, {"X"=1.11, "Y"=0.2154581617702197}, {"X"=1.12, "Y"=0.21306914677571784}, {"X"=1.13, "Y"=0.21068555173601533}, {"X"=1.14, "Y"=0.20830779004710837}, {"X"=1.15, "Y"=0.20593626871997478}, {"X"=1.16, "Y"=0.20357138829075944}, {"X"=1.17, "Y"=0.2012135427351974}, {"X"=1.18, "Y"=0.1988631193872759}, {"X"=1.19, "Y"=0.19652049886213654}, {"X"=1.2, "Y"=0.19418605498321298}, {"X"=1.21, "Y"=0.1918601547135994}, {"X"=1.22, "Y"=0.18954315809164027}, {"X"=1.23, "Y"=0.18723541817072956}, {"X"=1.24, "Y"=0.1849372809633053}, {"X"=1.25, "Y"=0.18264908538902191}, {"X"=1.26, "Y"=0.18037116322708033}, {"X"=1.27, "Y"=0.1781038390726936}, {"X"=1.28, "Y"=0.17584743029766237}, {"X"=1.29, "Y"=0.173602247015033}, {"X"=1.3, "Y"=0.17136859204780736}, {"X"=1.31, "Y"=0.1691467609016724}, {"X"=1.32, "Y"=0.1669370417417138}, {"X"=1.33, "Y"=0.1647397153730768}, {"X"=1.34, "Y"=0.16255505522553412}, {"X"=1.35, "Y"=0.1603833273419196}, {"X"=1.36, "Y"=0.15822479037038303}, {"X"=1.37, "Y"=0.15607969556042084}, {"X"=1.38, "Y"=0.15394828676263372}, {"X"=1.39, "Y"=0.1518308004321617}, {"X"=1.4, "Y"=0.14972746563574488}, {"X"=1.41, "Y"=0.14763850406235574}, {"X"=1.42, "Y"=0.1455641300373476}, {"X"=1.43, "Y"=0.14350455054006242}, {"X"=1.44, "Y"=0.1414599652248388}, {"X"=1.45, "Y"=0.13943056644536028}, {"X"=1.46, "Y"=0.13741653928228179}, {"X"=1.47, "Y"=0.1354180615740713}, {"X"=1.48, "Y"=0.13343530395100234}, {"X"=1.49, "Y"=0.13146842987223106}, {"X"=1.5, "Y"=0.12951759566589174}, {"X"=1.51, "Y"=0.12758295057214186}, {"X"=1.52, "Y"=0.12566463678908815}, {"X"=1.53, "Y"=0.12376278952152314}, {"X"=1.54, "Y"=0.12187753703240178}, {"X"=1.55, "Y"=0.12000900069698558}, {"X"=1.56, "Y"=0.11815729505958228}, {"X"=1.57, "Y"=0.1163225278928071}, {"X"=1.58, "Y"=0.11450480025929236}, {"X"=1.59, "Y"=0.11270420657577056}, {"X"=1.6, "Y"=0.11092083467945554}, {"X"=1.61, "Y"=0.10915476589664735}, {"X"=1.62, "Y"=0.1074060751134838}, {"X"=1.63, "Y"=0.10567483084876363}, {"X"=1.64, "Y"=0.10396109532876424}, {"X"=1.65, "Y"=0.10226492456397804}, {"X"=1.66, "Y"=0.10058636842769057}, {"X"=1.67, "Y"=0.09892547073632373}, {"X"=1.68, "Y"=0.09728226933146752}, {"X"=1.69, "Y"=0.09565679616352402}, {"X"=1.7, "Y"=0.09404907737688695}, {"X"=1.71, "Y"=0.09245913339658068}, {"X"=1.72, "Y"=0.09088697901628288}, {"X"=1.73, "Y"=0.089332623487655}, {"X"=1.74, "Y"=0.08779607061090564}, {"X"=1.75, "Y"=0.08627731882651153}, {"X"=1.76, "Y"=0.08477636130802224}, {"X"=1.77, "Y"=0.08329318605587446}, {"X"=1.78, "Y"=0.08182777599214282}, {"X"=1.79, "Y"=0.08038010905615417}, {"X"=1.8, "Y"=0.07895015830089415}, {"X"=1.81, "Y"=0.07753789199013399}, {"X"=1.82, "Y"=0.07614327369620731}, {"X"=1.83, "Y"=0.0747662623983676}, {"X"=1.84, "Y"=0.07340681258165689}, {"X"=1.85, "Y"=0.072064874336218}, {"X"=1.86, "Y"=0.07074039345698338}, {"X"=1.87, "Y"=0.06943331154367419}, {"X"=1.88, "Y"=0.06814356610104459}, {"X"=1.89, "Y"=0.06687109063930716}, {"X"=1.9, "Y"=0.0656158147746766}, {"X"=1.91, "Y"=0.06437766432996936}, {"X"=1.92, "Y"=0.06315656143519865}, {"X"=1.93, "Y"=0.061952424628105164}, {"X"=1.94, "Y"=0.06076516895456478}, {"X"=1.95, "Y"=0.059594706068816075}, {"X"=1.96, "Y"=0.058440944333451476}, {"X"=1.97, "Y"=0.05730378891911713}, {"X"=1.98, "Y"=0.05618314190386805}, {"X"=1.99, "Y"=0.05507890237212577}, {"X"=2.0, "Y"=0.05399096651318806}, {"X"=2.01, "Y"=0.05291922771924032}, {"X"=2.02, "Y"=0.051863576682820565}, {"X"=2.03, "Y"=0.05082390149369121}, {"X"=2.04, "Y"=0.049800087735070775}, {"X"=2.05, "Y"=0.04879201857918277}, {"X"=2.06, "Y"=0.047799574882077034}, {"X"=2.07, "Y"=0.04682263527768316}, {"X"=2.08, "Y"=0.045861076271054894}, {"X"=2.09, "Y"=0.0449147723307671}, {"X"=2.1, "Y"=0.0439835959804272}, {"X"=2.11, "Y"=0.04306741788926574}, {"X"=2.12, "Y"=0.04216610696177031}, {"X"=2.13, "Y"=0.041279530426330424}, {"X"=2.14, "Y"=0.04040755392286031}, {"X"=2.15, "Y"=0.03955004158937022}, {"X"=2.16, "Y"=0.03870685614745561}, {"X"=2.17, "Y"=0.03787785898667748}, {"X"=2.18, "Y"=0.037062910247806474}, {"X"=2.19, "Y"=0.03626186890490622}, {"X"=2.2, "Y"=0.035474592846231424}, {"X"=2.21, "Y"=0.03470093895391882}, {"X"=2.22, "Y"=0.033940763182449186}, {"X"=2.23, "Y"=0.03319392063586112}, {"X"=2.24, "Y"=0.032460265643697445}, {"X"=2.25, "Y"=0.03173965183566742}, {"X"=2.26, "Y"=0.031031932215008273}, {"X"=2.27, "Y"=0.03033695923053164}, {"X"=2.28, "Y"=0.029654584847341278}, {"X"=2.29, "Y"=0.028984660616209416}, {"X"=2.3, "Y"=0.02832703774160119}, {"X"=2.31, "Y"=0.027681567148336573}, {"X"=2.32, "Y"=0.027048099546881785}, {"X"=2.33, "Y"=0.026426485497261724}, {"X"=2.34, "Y"=0.02581657547158769}, {"X"=2.35, "Y"=0.025218219915194382}, {"X"=2.36, "Y"=0.024631269306382507}, {"X"=2.37, "Y"=0.02405557421476297}, {"X"=2.38, "Y"=0.023490985358201367}, {"X"=2.39, "Y"=0.022937353658360693}, {"X"=2.4, "Y"=0.0223945302948429}, {"X"=2.41, "Y"=0.021862366757929387}, {"X"=2.42, "Y"=0.021340714899922786}, {"X"=2.43, "Y"=0.020829426985092186}, {"X"=2.44, "Y"=0.02032835573822584}, {"X"=2.45, "Y"=0.019837354391795313}, {"X"=2.46, "Y"=0.019356276731736965}, {"X"=2.47, "Y"=0.018884977141856163}, {"X"=2.48, "Y"=0.01842331064686205}, {"X"=2.49, "Y"=0.017971132954039633}, {"X"=2.5, "Y"=0.01752830049356854}, {"X"=2.51, "Y"=0.017094670457496956}, {"X"=2.52, "Y"=0.016670100837381057}, {"X"=2.53, "Y"=0.016254450460600506}, {"X"=2.54, "Y"=0.015847579025360818}, {"X"=2.55, "Y"=0.015449347134395174}, {"X"=2.56, "Y"=0.01505961632737745}, {"X"=2.57, "Y"=0.014678249112060044}, {"X"=2.58, "Y"=0.014305108994149692}, {"X"=2.59, "Y"=0.013940060505935825}, {"X"=2.6, "Y"=0.013582969233685615}, {"X"=2.61, "Y"=0.013233701843821374}, {"X"=2.62, "Y"=0.012892126107895304}, {"X"=2.63, "Y"=0.012558110926378211}, {"X"=2.64, "Y"=0.012231526351277971}, {"X"=2.65, "Y"=0.01191224360760518}, {"X"=2.66, "Y"=0.011600135113702562}, {"X"=2.67, "Y"=0.011295074500456135}, {"X"=2.68, "Y"=0.010996936629405572}, {"X"=2.69, "Y"=0.010705597609772188}, {"X"=2.7, "Y"=0.010420934814422592}, {"X"=2.71, "Y"=0.010142826894787078}, {"X"=2.72, "Y"=0.009871153794751132}, {"X"=2.73, "Y"=0.009605796763539587}, {"X"=2.74, "Y"=0.009346638367612283}, {"X"=2.75, "Y"=0.009093562501591053}, {"X"=2.76, "Y"=0.008846454398237232}, {"X"=2.77, "Y"=0.008605200637499673}, {"X"=2.78, "Y"=0.008369689154653033}, {"X"=2.79, "Y"=0.008139809247546021}, {"X"=2.8, "Y"=0.007915451582979969}, {"X"=2.81, "Y"=0.007696508202237322}, {"X"=2.82, "Y"=0.007482872525780564}, {"X"=2.83, "Y"=0.007274439357141218}, {"X"=2.84, "Y"=0.007071104886019449}, {"X"=2.85, "Y"=0.006872766690613971}, {"X"=2.86, "Y"=0.00667932373920262}, {"X"=2.87, "Y"=0.006490676390993364}, {"X"=2.88, "Y"=0.0063067263962659275}, {"X"=2.89, "Y"=0.006127376895823688}, {"X"=2.9, "Y"=0.005952532419775854}, {"X"=2.91, "Y"=0.005782098885669473}, {"X"=2.92, "Y"=0.005615983595990969}, {"X"=2.93, "Y"=0.005454095235056545}, {"X"=2.94, "Y"=0.00529634386531102}, {"X"=2.95, "Y"=0.005142640923053939}, {"X"=2.96, "Y"=0.004992899213612376}, {"X"=2.97, "Y"=0.004847032905978945}, {"X"=2.98, "Y"=0.004704957526933979}, {"X"=2.99, "Y"=0.004566589954670145}, {"X"=3.0, "Y"=0.0044318484119380075}, {"X"=3.01, "Y"=0.00430065245873045}, {"X"=3.02, "Y"=0.004172922984523962}, {"X"=3.03, "Y"=0.00404858220009443}, {"X"=3.04, "Y"=0.003927553628924779}, {"X"=3.05, "Y"=0.0038097620982218104}, {"X"=3.06, "Y"=0.003695133729559035}, {"X"=3.07, "Y"=0.0035835959291623614}, {"X"=3.08, "Y"=0.003475077377854938}, {"X"=3.09, "Y"=0.0033695080206774812}, {"X"=3.1, "Y"=0.0032668190561999186}, {"X"=3.11, "Y"=0.0031669429255400815}, {"X"=3.12, "Y"=0.0030698133011047403}, {"X"=3.13, "Y"=0.002975365075068254}, {"X"=3.14, "Y"=0.002883534347603439}, {"X"=3.15, "Y"=0.002794258414879447}, {"X"=3.16, "Y"=0.0027074757568407003}, {"X"=3.17, "Y"=0.0026231260247810244}, {"X"=3.18, "Y"=0.002541150028726522}, {"X"=3.19, "Y"=0.0024614897246407006}, {"X"=3.2, "Y"=0.0023840882014648404}, {"X"=3.21, "Y"=0.0023088896680064958}, {"X"=3.22, "Y"=0.0022358394396885385}, {"X"=3.23, "Y"=0.0021648839251710624}, {"X"=3.24, "Y"=0.002095970612857942}, {"X"=3.25, "Y"=0.002029048057299768}, {"X"=3.26, "Y"=0.001964065865504376}, {"X"=3.27, "Y"=0.0019009746831660803}, {"X"=3.28, "Y"=0.0018397261808242812}, {"X"=3.29, "Y"=0.0017802730399618788}, {"X"=3.3, "Y"=0.0017225689390536812}, {"X"=3.31, "Y"=0.0016665685395745797}, {"X"=3.32, "Y"=0.0016122274719771244}, {"X"=3.33, "Y"=0.0015595023216476915}, {"X"=3.34, "Y"=0.0015083506148503075}, {"X"=3.35, "Y"=0.0014587308046667459}, {"X"=3.36, "Y"=0.001410602256941385}, {"X"=3.37, "Y"=0.0013639252362389036}, {"X"=3.38, "Y"=0.0013186608918227423}, {"X"=3.39, "Y"=0.001274771243661833}, {"X"=3.4, "Y"=0.00123221916847302}, {"X"=3.41, "Y"=0.0011909683858061168}, {"X"=3.42, "Y"=0.0011509834441784845}, {"X"=3.43, "Y"=0.0011122297072655649}, {"X"=3.44, "Y"=0.0010746733401537356}, {"X"=3.45, "Y"=0.0010382812956614103}, {"X"=3.46, "Y"=0.0010030213007342376}, {"X"=3.47, "Y"=0.0009688618429198459}, {"X"=3.48, "Y"=0.0009357721569274798}, {"X"=3.49, "Y"=0.0009037222112775245}, {"X"=3.5, "Y"=0.0008726826950457602}, {"X"=3.51, "Y"=0.0008426250047069028}, {"X"=3.52, "Y"=0.0008135212310818085}, {"X"=3.53, "Y"=0.00078534414639247}, {"X"=3.54, "Y"=0.0007580671914287103}, {"X"=3.55, "Y"=0.0007316644628303109}, {"X"=3.56, "Y"=0.0007061107004880362}, {"X"=3.57, "Y"=0.0006813812750668921}, {"X"=3.58, "Y"=0.0006574521756546766}, {"X"=3.59, "Y"=0.0006342999975387576}, {"X"=3.6, "Y"=0.0006119019301137719}, {"X"=3.61, "Y"=0.0005902357449227856}, {"X"=3.62, "Y"=0.0005692797838342526}, {"X"=3.63, "Y"=0.0005490129473569587}, {"X"=3.64, "Y"=0.0005294146830949348}, {"X"=3.65, "Y"=0.0005104649743441856}, {"X"=3.66, "Y"=0.0004921443288328931}, {"X"=3.67, "Y"=0.00047443376760662064}, {"X"=3.68, "Y"=0.00045731481405985675}, {"X"=3.69, "Y"=0.0004407694831151325}, {"X"=3.7, "Y"=0.00042478027055075143}, {"X"=3.71, "Y"=0.0004093301424780789}, {"X"=3.72, "Y"=0.0003944025249691562}, {"X"=3.73, "Y"=0.00037998129383532146}, {"X"=3.74, "Y"=0.000366050764557335}, {"X"=3.75, "Y"=0.00035259568236744546}, {"X"=3.76, "Y"=0.0003396012124836548}, {"X"=3.77, "Y"=0.00032705293049637503}, {"X"=3.78, "Y"=0.0003149368129075219}, {"X"=3.79, "Y"=0.0003032392278220042}, {"X"=3.8, "Y"=0.00029194692579146027}, {"X"=3.81, "Y"=0.0002810470308099863}, {"X"=3.82, "Y"=0.000270527031461521}, {"X"=3.83, "Y"=0.00026037477221844247}, {"X"=3.84, "Y"=0.00025057844489086075}, {"X"=3.85, "Y"=0.00024112658022599324}, {"X"=3.86, "Y"=0.00023200803965694238}, {"X"=3.87, "Y"=0.0002232120072001021}, {"X"=3.88, "Y"=0.00021472798150036704}, {"X"=3.89, "Y"=0.00020654576802322548}, {"X"=3.9, "Y"=0.00019865547139277272}, {"X"=3.91, "Y"=0.00019104748787459762}, {"X"=3.92, "Y"=0.0001837124980024571}, {"X"=3.93, "Y"=0.00017664145934757092}, {"X"=3.94, "Y"=0.00016982559942934359}, {"X"=3.95, "Y"=0.00016325640876624202}, {"X"=3.96, "Y"=0.00015692563406553226}, {"X"=3.97, "Y"=0.0001508252715505178}, {"X"=3.98, "Y"=0.00014494756042389106}, {"X"=3.99, "Y"=0.00013928497646575994}, {"X"=4.0, "Y"=0.00013383022576488537}, {"X"=4.01, "Y"=0.00012857623858162108}, {"X"=4.02, "Y"=0.00012351616334102368}, {"X"=4.03, "Y"=0.00011864336075456578}, {"X"=4.04, "Y"=0.00011395139806886461}, {"X"=4.05, "Y"=0.00010943404343980055}, {"X"=4.06, "Y"=0.00010508526043040049}, {"X"=4.07, "Y"=0.00010089920263081443}, {"X"=4.08, "Y"=9.687020839871927e-05}, {"X"=4.09, "Y"=9.299279571844591e-05}, {"X"=4.1, "Y"=8.926165717713293e-05}, {"X"=4.11, "Y"=8.567165505618186e-05}, {"X"=4.12, "Y"=8.2217816536286e-05}, {"X"=4.13, "Y"=7.889532901429309e-05}, {"X"=4.14, "Y"=7.569953553016121e-05}, {"X"=4.15, "Y"=7.262593030225234e-05}, {"X"=4.16, "Y"=6.967015436921434e-05}, {"X"=4.17, "Y"=6.682799133669061e-05}, {"X"=4.18, "Y"=6.40953632271061e-05}, {"X"=4.19, "Y"=6.146832643076922e-05}, {"X"=4.2, "Y"=5.8943067756539855e-05}, {"X"=4.21, "Y"=5.651590058030741e-05}, {"X"=4.22, "Y"=5.4183261089540144e-05}, {"X"=4.23, "Y"=5.1941704622159776e-05}, {"X"=4.24, "Y"=4.978790209801209e-05}, {"X"=4.25, "Y"=4.771863654120495e-05}, {"X"=4.26, "Y"=4.5730799691601314e-05}, {"X"=4.27, "Y"=4.382138870375812e-05}, {"X"=4.28, "Y"=4.198750293161732e-05}, {"X"=4.29, "Y"=4.022634079726497e-05}, {"X"=4.3, "Y"=3.853519674208713e-05}, {"X"=4.31, "Y"=3.69114582586662e-05}, {"X"=4.32, "Y"=3.5352603001773097e-05}, {"X"=4.33, "Y"=3.385619597682789e-05}, {"X"=4.34, "Y"=3.241988680421378e-05}, {"X"=4.35, "Y"=3.1041407057850266e-05}, {"X"=4.36, "Y"=2.97185676764422e-05}, {"X"=4.37, "Y"=2.8449256445844308e-05}, {"X"=4.38, "Y"=2.723143555099261e-05}, {"X"=4.39, "Y"=2.6063139195878346e-05}, {"X"=4.4, "Y"=2.4942471290053535e-05}, {"X"=4.41, "Y"=2.38676032001796e-05}, {"X"=4.42, "Y"=2.283677156514692e-05}, {"X"=4.43, "Y"=2.184827617331647e-05}, {"X"=4.44, "Y"=2.0900477900450407e-05}, {"X"=4.45, "Y"=1.999179670692279e-05}, {"X"=4.46, "Y"=1.9120709692817737e-05}, {"X"=4.47, "Y"=1.828574920954738e-05}, {"X"=4.48, "Y"=1.748550102663914e-05}, {"X"=4.49, "Y"=1.671860255236507e-05}, {"X"=4.5, "Y"=1.5983741106905478e-05}, {"X"=4.51, "Y"=1.527965224676162e-05}, {"X"=4.52, "Y"=1.4605118139152942e-05}, {"X"=4.53, "Y"=1.3958965985154772e-05}, {"X"=4.54, "Y"=1.334006649035584e-05}, {"X"=4.55, "Y"=1.2747332381833467e-05}, {"X"=4.56, "Y"=1.21797169702687e-05}, {"X"=4.57, "Y"=1.1636212756042669e-05}, {"X"=4.58, "Y"=1.111585007817779e-05}, {"X"=4.59, "Y"=1.0617695805008393e-05}, {"X"=4.6, "Y"=1.014085206548676e-05}, {"X"=4.61, "Y"=9.684455020051437e-06}, {"X"=4.62, "Y"=9.247673670005617e-06}, {"X"=4.63, "Y"=8.829708704374098e-06}, {"X"=4.64, "Y"=8.429791383228772e-06}, {"X"=4.65, "Y"=8.047182456492295e-06}, {"X"=4.66, "Y"=7.681171117250455e-06}, {"X"=4.67, "Y"=7.331073988623946e-06}, {"X"=4.68, "Y"=6.996234143270405e-06}, {"X"=4.69, "Y"=6.676020154607462e-06}, {"X"=4.7, "Y"=6.36982517886709e-06}, {"X"=4.71, "Y"=6.077066067111116e-06}, {"X"=4.72, "Y"=5.797182506357288e-06}, {"X"=4.73, "Y"=5.529636188984052e-06}, {"X"=4.74, "Y"=5.273910009601304e-06}, {"X"=4.75, "Y"=5.029507288592446e-06}, {"X"=4.76, "Y"=4.795951021552522e-06}, {"X"=4.77, "Y"=4.5727831538641446e-06}, {"X"=4.78, "Y"=4.359563879671637e-06}, {"X"=4.79, "Y"=4.155870964531201e-06}, {"X"=4.8, "Y"=3.961299091032075e-06}, {"X"=4.81, "Y"=3.775459226701349e-06}, {"X"=4.82, "Y"=3.5979780135212474e-06}, {"X"=4.83, "Y"=3.428497178405039e-06}, {"X"=4.84, "Y"=3.266672963993275e-06}, {"X"=4.85, "Y"=3.112175579148945e-06}, {"X"=4.86, "Y"=2.964688668545273e-06}, {"X"=4.87, "Y"=2.823908800755821e-06}, {"X"=4.88, "Y"=2.6895449742715237e-06}, {"X"=4.89, "Y"=2.5613181408845447e-06}, {"X"=4.9, "Y"=2.438960745893352e-06}, {"X"=4.91, "Y"=2.322216284597997e-06}, {"X"=4.92, "Y"=2.2108388745684212e-06}, {"X"=4.93, "Y"=2.10459284318313e-06}, {"X"=4.94, "Y"=2.0032523299484894e-06}, {"X"=4.95, "Y"=1.906600903122811e-06}, {"X"=4.96, "Y"=1.8144311901820306e-06}, {"X"=4.97, "Y"=1.7265445216770736e-06}, {"X"=4.98, "Y"=1.6427505880450713e-06}, {"X"=4.99, "Y"=1.5628671089492902e-06}, {"X"=5.0, "Y"=1.4867195147342979e-06}, {"X"=5.01, "Y"=1.4141406395950037e-06}, {"X"=5.02, "Y"=1.3449704260694445e-06}, {"X"=5.03, "Y"=1.2790556404765742e-06}, {"X"=5.04, "Y"=1.216249598931318e-06}, {"X"=5.05, "Y"=1.1564119035797834e-06}, {"X"=5.06, "Y"=1.0994081887082052e-06}, {"X"=5.07, "Y"=1.0451098763893177e-06}, {"X"=5.08, "Y"=9.93393941339912e-07}, {"X"=5.09, "Y"=9.441426846730874e-07}, {"X"=5.1, "Y"=8.972435162383337e-07}, {"X"=5.11, "Y"=8.52588745251786e-07}, {"X"=5.12, "Y"=8.100753789281346e-07}, {"X"=5.13, "Y"=7.696049288345129e-07}, {"X"=5.14, "Y"=7.310832246953503e-07}, {"X"=5.15, "Y"=6.944202353855339e-07}, {"X"=5.16, "Y"=6.595298968575217e-07}, {"X"=5.17, "Y"=6.263299467558902e-07}, {"X"=5.18, "Y"=5.947417654807764e-07}, {"X"=5.19, "Y"=5.64690223469076e-07}, {"X"=5.2, "Y"=5.361035344697615e-07}, {"X"=5.21, "Y"=5.08913114596766e-07}, {"X"=5.22, "Y"=4.830534469499683e-07}, {"X"=5.23, "Y"=4.584619516015329e-07}, {"X"=5.24, "Y"=4.350788607515109e-07}, {"X"=5.25, "Y"=4.1284709886299984e-07}, {"X"=5.26, "Y"=3.9171216759348166e-07}, {"X"=5.27, "Y"=3.7162203534495063e-07}, {"X"=5.28, "Y"=3.525270312614038e-07}, {"X"=5.29, "Y"=3.3437974350798003e-07}, {"X"=5.3, "Y"=3.171349216715976e-07}, {"X"=5.31, "Y"=3.007493831283838e-07}, {"X"=5.32, "Y"=2.851819232283976e-07}, {"X"=5.33, "Y"=2.7039322915329305e-07}, {"X"=5.34, "Y"=2.5634579730745934e-07}, {"X"=5.35, "Y"=2.4300385410805355e-07}, {"X"=5.36, "Y"=2.3033328004392066e-07}, {"X"=5.37, "Y"=2.1830153687797888e-07}, {"X"=5.38, "Y"=2.0687759787196552e-07}, {"X"=5.39, "Y"=1.9603188091675758e-07}, {"X"=5.4, "Y"=1.8573618445552897e-07}, {"X"=5.41, "Y"=1.7596362609104592e-07}, {"X"=5.42, "Y"=1.6668858377222828e-07}, {"X"=5.43, "Y"=1.5788663945889064e-07}, {"X"=5.44, "Y"=1.495345251671592e-07}, {"X"=5.45, "Y"=1.4161007130161178e-07}, {"X"=5.46, "Y"=1.3409215718354753e-07}, {"X"=5.47, "Y"=1.2696066368812932e-07}, {"X"=5.48, "Y"=1.201964279062823e-07}, {"X"=5.49, "Y"=1.1378119975034591e-07}, {"X"=5.5, "Y"=1.0769760042543276e-07}, {"X"=5.51, "Y"=1.0192908269135293e-07}, {"X"=5.52, "Y"=9.645989284273384e-08}, {"X"=5.53, "Y"=9.127503433766477e-08}, {"X"=5.54, "Y"=8.636023300780988e-08}, {"X"=5.55, "Y"=8.17019037854322e-08}, {"X"=5.56, "Y"=7.728711888522921e-08}, {"X"=5.57, "Y"=7.310357738120935e-08}, {"X"=5.58, "Y"=6.913957612112398e-08}, {"X"=5.59, "Y"=6.538398192315145e-08}, {"X"=5.6, "Y"=6.182620500165857e-08}, {"X"=5.61, "Y"=5.84561735709005e-08}, {"X"=5.62, "Y"=5.526430957749716e-08}, {"X"=5.63, "Y"=5.2241505514424374e-08}, {"X"=5.64, "Y"=4.937910227110449e-08}, {"X"=5.65, "Y"=4.666886797594257e-08}, {"X"=5.66, "Y"=4.410297778937308e-08}, {"X"=5.67, "Y"=4.167399460712351e-08}, {"X"=5.68, "Y"=3.9374850634998504e-08}, {"X"=5.69, "Y"=3.7198829798016034e-08}, {"X"=5.7, "Y"=3.513955094820434e-08}, {"X"=5.71, "Y"=3.319095183679538e-08}, {"X"=5.72, "Y"=3.134727381791979e-08}, {"X"=5.73, "Y"=2.960304725223005e-08}, {"X"=5.74, "Y"=2.795307758015465e-08}, {"X"=5.75, "Y"=2.6392432035705735e-08}, {"X"=5.76, "Y"=2.4916426972950992e-08}, {"X"=5.77, "Y"=2.352061577839084e-08}, {"X"=5.78, "Y"=2.2200777343579013e-08}, {"X"=5.79, "Y"=2.0952905073377047e-08}, {"X"=5.8, "Y"=1.9773196406244675e-08}, {"X"=5.81, "Y"=1.865804282394618e-08}, {"X"=5.82, "Y"=1.7604020328985783e-08}, {"X"=5.83, "Y"=1.6607880368992047e-08}, {"X"=5.84, "Y"=1.5666541188132572e-08}, {"X"=5.85, "Y"=1.4777079586480055e-08}, {"X"=5.86, "Y"=1.3936723069047392e-08}, {"X"=5.87, "Y"=1.3142842366982143e-08}, {"X"=5.88, "Y"=1.239294431415013e-08}, {"X"=5.89, "Y"=1.168466506304987e-08}, {"X"=5.9, "Y"=1.1015763624682308e-08}, {"X"=5.91, "Y"=1.0384115717656327e-08}, {"X"=5.92, "Y"=9.78770791244118e-09}, {"X"=5.93, "Y"=9.22463205728272e-09}, {"X"=5.94, "Y"=8.693079972880173e-09}, {"X"=5.95, "Y"=8.191338403479174e-09}, {"X"=5.96, "Y"=7.717784212570529e-09}, {"X"=5.97, "Y"=7.270879811900108e-09}, {"X"=5.98, "Y"=6.8491688129857586e-09}, {"X"=5.99, "Y"=6.451271890811751e-09}, {"X"=6.0, "Y"=6.075882849823286e-09}, {"X"=6.01, "Y"=5.7217648827798965e-09}, {"X"=6.02, "Y"=5.38774701344276e-09}, {"X"=6.03, "Y"=5.072720714470481e-09}, {"X"=6.04, "Y"=4.775636692282276e-09}, {"X"=6.05, "Y"=4.4955018310132455e-09}, {"X"=6.06, "Y"=4.231376288039894e-09}, {"X"=6.07, "Y"=3.982370733890178e-09}, {"X"=6.08, "Y"=3.747643729676039e-09}, {"X"=6.09, "Y"=3.526399235495381e-09}]
  # "NORMAL DISTRIBUTION"
  # "NORMAL DISTRIBUTION"
  # "Standard Normal Distribution"
  # "Standard Normal Distribution"
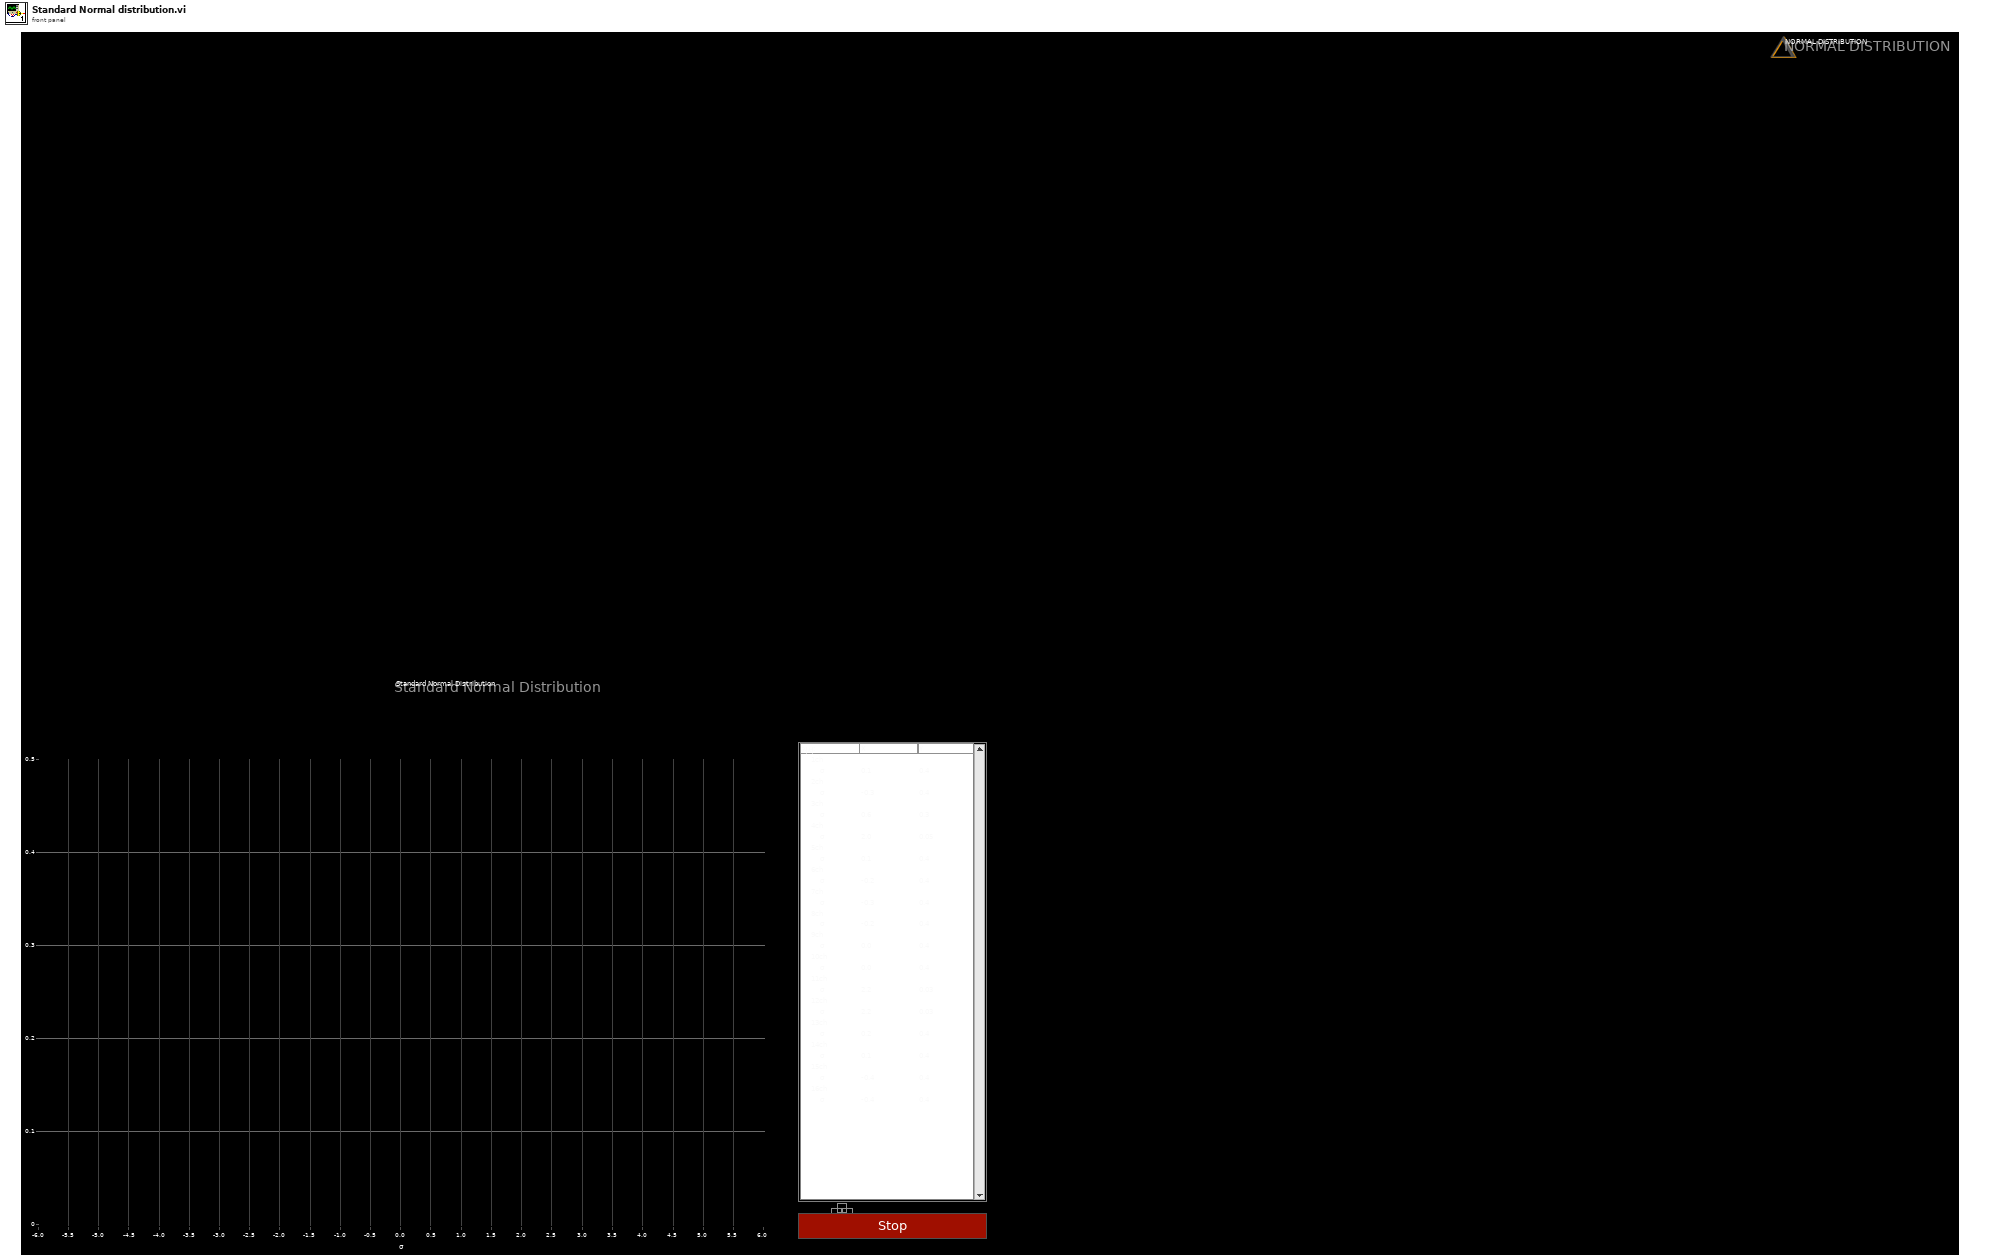
[diagram p1: front panel]
types:
  T1 = cluster{"Name":string, "Color":u32, "Style":u8, "Point Style":u8, "Name Visible":bool, "Allow Drag":bool, "Cursor Mode":u32, "Plot":i32, "Index":i32, "Position":cluster{"X":dbl, "Y":dbl}, "X Scale":u32, "Y Scale":u32, "Watch Plots":i32[], "Watch All Plots":bool, "Plot Area":i32, "Label Offset":cluster{"X":dbl, "Y":dbl}}
  T2 = enum16{"arithmetic", "geometric", "harmonic", "trimmed", "median"}
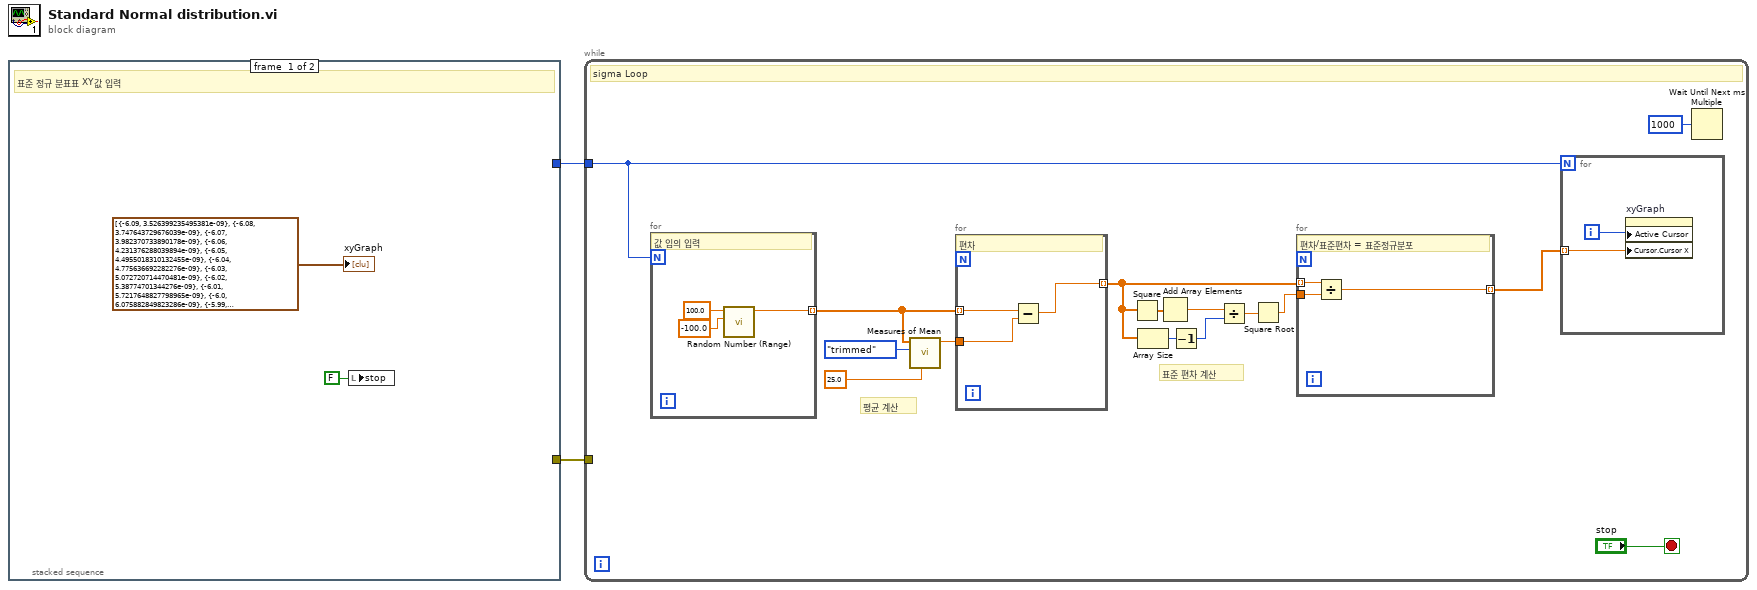
[diagram p0: block diagram]
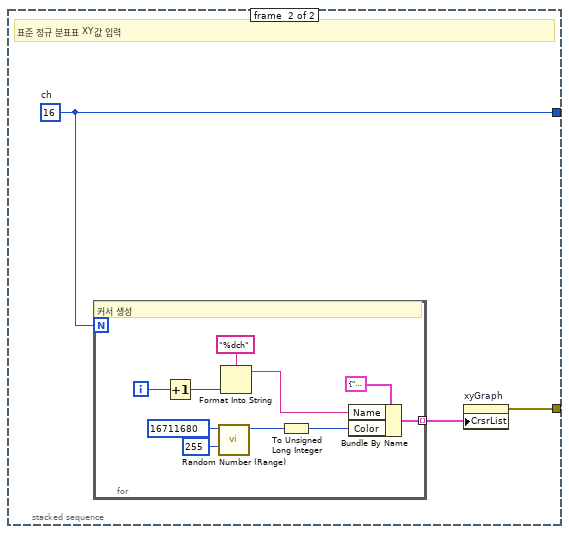
[diagram p2: hidden frame]
diagram:
  n1 = stacked-sequence {
    tunnel: [_ w6] -> w2
    tunnel: [_ w5] -> w1
    frame #0 {
      # "표준 정규 분표표 XY값 입력"
      n2 = local write "stop"(FALSE ("stop")) -> ()
      "xyGraph" <- cluster{"X":dbl, "Y":dbl}[] [{"X"=-6.09, "Y"=3.526399235495381e-09}, {"X"=-6.08, "Y"=3.747643729676039e-09}, {"X"=-6.07, "Y"=3.982370733890178e-09}, {"X"=-6.06, "Y"=4.231376288039894e-09}, {"X"=-6.05, "Y"=4.4955018310132455e-09}, {"X"=-6.04, "Y"=4.775636692282276e-09}, {"X"=-6.03, "Y"=5.072720714470481e-09}, {"X"=-6.02, "Y"=5.38774701344276e-09}, {"X"=-6.01, "Y"=5.7217648827798965e-09}, {"X"=-6.0, "Y"=6.075882849823286e-09}, {"X"=-5.99, "Y"=6.451271890811751e-09}, {"X"=-5.98, "Y"=6.8491688129857586e-09}, {"X"=-5.97, "Y"=7.270879811900108e-09}, {"X"=-5.96, "Y"=7.717784212570529e-09}, {"X"=-5.95, "Y"=8.191338403479174e-09}, {"X"=-5.94, "Y"=8.693079972880173e-09}, {"X"=-5.93, "Y"=9.22463205728272e-09}, {"X"=-5.92, "Y"=9.78770791244118e-09}, {"X"=-5.91, "Y"=1.0384115717656327e-08}, {"X"=-5.9, "Y"=1.1015763624682308e-08}, {"X"=-5.89, "Y"=1.168466506304987e-08}, {"X"=-5.88, "Y"=1.239294431415013e-08}, {"X"=-5.87, "Y"=1.3142842366982143e-08}, {"X"=-5.86, "Y"=1.3936723069047392e-08}, {"X"=-5.85, "Y"=1.4777079586480055e-08}, {"X"=-5.84, "Y"=1.5666541188132572e-08}, {"X"=-5.83, "Y"=1.6607880368992047e-08}, {"X"=-5.82, "Y"=1.7604020328985783e-08}, {"X"=-5.81, "Y"=1.865804282394618e-08}, {"X"=-5.8, "Y"=1.9773196406244675e-08}, {"X"=-5.79, "Y"=2.0952905073377047e-08}, {"X"=-5.78, "Y"=2.2200777343579013e-08}, {"X"=-5.77, "Y"=2.352061577839084e-08}, {"X"=-5.76, "Y"=2.4916426972950992e-08}, {"X"=-5.75, "Y"=2.6392432035705735e-08}, {"X"=-5.74, "Y"=2.795307758015465e-08}, {"X"=-5.73, "Y"=2.960304725223005e-08}, {"X"=-5.72, "Y"=3.134727381791979e-08}, {"X"=-5.71, "Y"=3.319095183679538e-08}, {"X"=-5.7, "Y"=3.513955094820434e-08}, {"X"=-5.69, "Y"=3.7198829798016034e-08}, {"X"=-5.68, "Y"=3.9374850634998504e-08}, {"X"=-5.67, "Y"=4.167399460712351e-08}, {"X"=-5.66, "Y"=4.410297778937308e-08}, {"X"=-5.65, "Y"=4.666886797594257e-08}, {"X"=-5.64, "Y"=4.937910227110449e-08}, {"X"=-5.63, "Y"=5.2241505514424374e-08}, {"X"=-5.62, "Y"=5.526430957749716e-08}, {"X"=-5.61, "Y"=5.84561735709005e-08}, {"X"=-5.6, "Y"=6.182620500165857e-08}, {"X"=-5.59, "Y"=6.538398192315145e-08}, {"X"=-5.58, "Y"=6.913957612112398e-08}, {"X"=-5.57, "Y"=7.310357738120935e-08}, {"X"=-5.56, "Y"=7.728711888522921e-08}, {"X"=-5.55, "Y"=8.17019037854322e-08}, {"X"=-5.54, "Y"=8.636023300780988e-08}, {"X"=-5.53, "Y"=9.127503433766477e-08}, {"X"=-5.52, "Y"=9.645989284273384e-08}, {"X"=-5.51, "Y"=1.0192908269135293e-07}, {"X"=-5.5, "Y"=1.0769760042543276e-07}, {"X"=-5.49, "Y"=1.1378119975034591e-07}, {"X"=-5.48, "Y"=1.201964279062823e-07}, {"X"=-5.47, "Y"=1.2696066368812932e-07}, {"X"=-5.46, "Y"=1.3409215718354753e-07}, {"X"=-5.45, "Y"=1.4161007130161178e-07}, {"X"=-5.44, "Y"=1.495345251671592e-07}, {"X"=-5.43, "Y"=1.5788663945889064e-07}, {"X"=-5.42, "Y"=1.6668858377222828e-07}, {"X"=-5.41, "Y"=1.7596362609104592e-07}, {"X"=-5.4, "Y"=1.8573618445552897e-07}, {"X"=-5.39, "Y"=1.9603188091675758e-07}, {"X"=-5.38, "Y"=2.0687759787196552e-07}, {"X"=-5.37, "Y"=2.1830153687797888e-07}, {"X"=-5.36, "Y"=2.3033328004392066e-07}, {"X"=-5.35, "Y"=2.4300385410805355e-07}, {"X"=-5.34, "Y"=2.5634579730745934e-07}, {"X"=-5.33, "Y"=2.7039322915329305e-07}, {"X"=-5.32, "Y"=2.851819232283976e-07}, {"X"=-5.31, "Y"=3.007493831283838e-07}, {"X"=-5.3, "Y"=3.171349216715976e-07}, {"X"=-5.29, "Y"=3.3437974350798003e-07}, {"X"=-5.28, "Y"=3.525270312614038e-07}, {"X"=-5.27, "Y"=3.7162203534495063e-07}, {"X"=-5.26, "Y"=3.9171216759348166e-07}, {"X"=-5.25, "Y"=4.1284709886299984e-07}, {"X"=-5.24, "Y"=4.350788607515109e-07}, {"X"=-5.23, "Y"=4.584619516015329e-07}, {"X"=-5.22, "Y"=4.830534469499683e-07}, {"X"=-5.21, "Y"=5.08913114596766e-07}, {"X"=-5.2, "Y"=5.361035344697615e-07}, {"X"=-5.19, "Y"=5.64690223469076e-07}, {"X"=-5.18, "Y"=5.947417654807764e-07}, {"X"=-5.17, "Y"=6.263299467558902e-07}, {"X"=-5.16, "Y"=6.595298968575217e-07}, {"X"=-5.15, "Y"=6.944202353855339e-07}, {"X"=-5.14, "Y"=7.310832246953503e-07}, {"X"=-5.13, "Y"=7.696049288345129e-07}, {"X"=-5.12, "Y"=8.100753789281346e-07}, {"X"=-5.11, "Y"=8.52588745251786e-07}, {"X"=-5.1, "Y"=8.972435162383337e-07}, {"X"=-5.09, "Y"=9.441426846730874e-07}, {"X"=-5.08, "Y"=9.93393941339912e-07}, {"X"=-5.07, "Y"=1.0451098763893177e-06}, {"X"=-5.06, "Y"=1.0994081887082052e-06}, {"X"=-5.05, "Y"=1.1564119035797834e-06}, {"X"=-5.04, "Y"=1.216249598931318e-06}, {"X"=-5.03, "Y"=1.2790556404765742e-06}, {"X"=-5.02, "Y"=1.3449704260694445e-06}, {"X"=-5.01, "Y"=1.4141406395950037e-06}, {"X"=-5.0, "Y"=1.4867195147342979e-06}, {"X"=-4.99, "Y"=1.5628671089492902e-06}, {"X"=-4.98, "Y"=1.6427505880450713e-06}, {"X"=-4.97, "Y"=1.7265445216770736e-06}, {"X"=-4.96, "Y"=1.8144311901820306e-06}, {"X"=-4.95, "Y"=1.906600903122811e-06}, {"X"=-4.94, "Y"=2.0032523299484894e-06}, {"X"=-4.93, "Y"=2.10459284318313e-06}, {"X"=-4.92, "Y"=2.2108388745684212e-06}, {"X"=-4.91, "Y"=2.322216284597997e-06}, {"X"=-4.9, "Y"=2.438960745893352e-06}, {"X"=-4.89, "Y"=2.5613181408845447e-06}, {"X"=-4.88, "Y"=2.6895449742715237e-06}, {"X"=-4.87, "Y"=2.823908800755821e-06}, {"X"=-4.86, "Y"=2.964688668545273e-06}, {"X"=-4.85, "Y"=3.112175579148945e-06}, {"X"=-4.84, "Y"=3.266672963993275e-06}, {"X"=-4.83, "Y"=3.428497178405039e-06}, {"X"=-4.82, "Y"=3.5979780135212474e-06}, {"X"=-4.81, "Y"=3.775459226701349e-06}, {"X"=-4.8, "Y"=3.961299091032075e-06}, {"X"=-4.79, "Y"=4.155870964531201e-06}, {"X"=-4.78, "Y"=4.359563879671637e-06}, {"X"=-4.77, "Y"=4.5727831538641446e-06}, {"X"=-4.76, "Y"=4.795951021552522e-06}, {"X"=-4.75, "Y"=5.029507288592446e-06}, {"X"=-4.74, "Y"=5.273910009601304e-06}, {"X"=-4.73, "Y"=5.529636188984052e-06}, {"X"=-4.72, "Y"=5.797182506357288e-06}, {"X"=-4.71, "Y"=6.077066067111116e-06}, {"X"=-4.7, "Y"=6.36982517886709e-06}, {"X"=-4.69, "Y"=6.676020154607462e-06}, {"X"=-4.68, "Y"=6.996234143270405e-06}, {"X"=-4.67, "Y"=7.331073988623946e-06}, {"X"=-4.66, "Y"=7.681171117250455e-06}, {"X"=-4.65, "Y"=8.047182456492295e-06}, {"X"=-4.64, "Y"=8.429791383228772e-06}, {"X"=-4.63, "Y"=8.829708704374098e-06}, {"X"=-4.62, "Y"=9.247673670005617e-06}, {"X"=-4.61, "Y"=9.684455020051437e-06}, {"X"=-4.6, "Y"=1.014085206548676e-05}, {"X"=-4.59, "Y"=1.0617695805008393e-05}, {"X"=-4.58, "Y"=1.111585007817779e-05}, {"X"=-4.57, "Y"=1.1636212756042669e-05}, {"X"=-4.56, "Y"=1.21797169702687e-05}, {"X"=-4.55, "Y"=1.2747332381833467e-05}, {"X"=-4.54, "Y"=1.334006649035584e-05}, {"X"=-4.53, "Y"=1.3958965985154772e-05}, {"X"=-4.52, "Y"=1.4605118139152942e-05}, {"X"=-4.51, "Y"=1.527965224676162e-05}, {"X"=-4.5, "Y"=1.5983741106905478e-05}, {"X"=-4.49, "Y"=1.671860255236507e-05}, {"X"=-4.48, "Y"=1.748550102663914e-05}, {"X"=-4.47, "Y"=1.828574920954738e-05}, {"X"=-4.46, "Y"=1.9120709692817737e-05}, {"X"=-4.45, "Y"=1.999179670692279e-05}, {"X"=-4.44, "Y"=2.0900477900450407e-05}, {"X"=-4.43, "Y"=2.184827617331647e-05}, {"X"=-4.42, "Y"=2.283677156514692e-05}, {"X"=-4.41, "Y"=2.38676032001796e-05}, {"X"=-4.4, "Y"=2.4942471290053535e-05}, {"X"=-4.39, "Y"=2.6063139195878346e-05}, {"X"=-4.38, "Y"=2.723143555099261e-05}, {"X"=-4.37, "Y"=2.8449256445844308e-05}, {"X"=-4.36, "Y"=2.97185676764422e-05}, {"X"=-4.35, "Y"=3.1041407057850266e-05}, {"X"=-4.34, "Y"=3.241988680421378e-05}, {"X"=-4.33, "Y"=3.385619597682789e-05}, {"X"=-4.32, "Y"=3.5352603001773097e-05}, {"X"=-4.31, "Y"=3.69114582586662e-05}, {"X"=-4.3, "Y"=3.853519674208713e-05}, {"X"=-4.29, "Y"=4.022634079726497e-05}, {"X"=-4.28, "Y"=4.198750293161732e-05}, {"X"=-4.27, "Y"=4.382138870375812e-05}, {"X"=-4.26, "Y"=4.5730799691601314e-05}, {"X"=-4.25, "Y"=4.771863654120495e-05}, {"X"=-4.24, "Y"=4.978790209801209e-05}, {"X"=-4.23, "Y"=5.1941704622159776e-05}, {"X"=-4.22, "Y"=5.4183261089540144e-05}, {"X"=-4.21, "Y"=5.651590058030741e-05}, {"X"=-4.2, "Y"=5.8943067756539855e-05}, {"X"=-4.19, "Y"=6.146832643076922e-05}, {"X"=-4.18, "Y"=6.40953632271061e-05}, {"X"=-4.17, "Y"=6.682799133669061e-05}, {"X"=-4.16, "Y"=6.967015436921434e-05}, {"X"=-4.15, "Y"=7.262593030225234e-05}, {"X"=-4.14, "Y"=7.569953553016121e-05}, {"X"=-4.13, "Y"=7.889532901429309e-05}, {"X"=-4.12, "Y"=8.2217816536286e-05}, {"X"=-4.11, "Y"=8.567165505618186e-05}, {"X"=-4.1, "Y"=8.926165717713293e-05}, {"X"=-4.09, "Y"=9.299279571844591e-05}, {"X"=-4.08, "Y"=9.687020839871927e-05}, {"X"=-4.07, "Y"=0.00010089920263081443}, {"X"=-4.06, "Y"=0.00010508526043040049}, {"X"=-4.05, "Y"=0.00010943404343980055}, {"X"=-4.04, "Y"=0.00011395139806886461}, {"X"=-4.03, "Y"=0.00011864336075456578}, {"X"=-4.02, "Y"=0.00012351616334102368}, {"X"=-4.01, "Y"=0.00012857623858162108}, {"X"=-4.0, "Y"=0.00013383022576488537}, {"X"=-3.99, "Y"=0.00013928497646575994}, {"X"=-3.98, "Y"=0.00014494756042389106}, {"X"=-3.97, "Y"=0.0001508252715505178}, {"X"=-3.96, "Y"=0.00015692563406553226}, {"X"=-3.95, "Y"=0.00016325640876624202}, {"X"=-3.94, "Y"=0.00016982559942934359}, {"X"=-3.93, "Y"=0.00017664145934757092}, {"X"=-3.92, "Y"=0.0001837124980024571}, {"X"=-3.91, "Y"=0.00019104748787459762}, {"X"=-3.9, "Y"=0.00019865547139277272}, {"X"=-3.89, "Y"=0.00020654576802322548}, {"X"=-3.88, "Y"=0.00021472798150036704}, {"X"=-3.87, "Y"=0.0002232120072001021}, {"X"=-3.86, "Y"=0.00023200803965694238}, {"X"=-3.85, "Y"=0.00024112658022599324}, {"X"=-3.84, "Y"=0.00025057844489086075}, {"X"=-3.83, "Y"=0.00026037477221844247}, {"X"=-3.82, "Y"=0.000270527031461521}, {"X"=-3.81, "Y"=0.0002810470308099863}, {"X"=-3.8, "Y"=0.00029194692579146027}, {"X"=-3.79, "Y"=0.0003032392278220042}, {"X"=-3.78, "Y"=0.0003149368129075219}, {"X"=-3.77, "Y"=0.00032705293049637503}, {"X"=-3.76, "Y"=0.0003396012124836548}, {"X"=-3.75, "Y"=0.00035259568236744546}, {"X"=-3.74, "Y"=0.000366050764557335}, {"X"=-3.73, "Y"=0.00037998129383532146}, {"X"=-3.72, "Y"=0.0003944025249691562}, {"X"=-3.71, "Y"=0.0004093301424780789}, {"X"=-3.7, "Y"=0.00042478027055075143}, {"X"=-3.69, "Y"=0.0004407694831151325}, {"X"=-3.68, "Y"=0.00045731481405985675}, {"X"=-3.67, "Y"=0.00047443376760662064}, {"X"=-3.66, "Y"=0.0004921443288328931}, {"X"=-3.65, "Y"=0.0005104649743441856}, {"X"=-3.64, "Y"=0.0005294146830949348}, {"X"=-3.63, "Y"=0.0005490129473569587}, {"X"=-3.62, "Y"=0.0005692797838342526}, {"X"=-3.61, "Y"=0.0005902357449227856}, {"X"=-3.6, "Y"=0.0006119019301137719}, {"X"=-3.59, "Y"=0.0006342999975387576}, {"X"=-3.58, "Y"=0.0006574521756546766}, {"X"=-3.57, "Y"=0.0006813812750668921}, {"X"=-3.56, "Y"=0.0007061107004880362}, {"X"=-3.55, "Y"=0.0007316644628303109}, {"X"=-3.54, "Y"=0.0007580671914287103}, {"X"=-3.53, "Y"=0.00078534414639247}, {"X"=-3.52, "Y"=0.0008135212310818085}, {"X"=-3.51, "Y"=0.0008426250047069028}, {"X"=-3.5, "Y"=0.0008726826950457602}, {"X"=-3.49, "Y"=0.0009037222112775245}, {"X"=-3.48, "Y"=0.0009357721569274798}, {"X"=-3.47, "Y"=0.0009688618429198459}, {"X"=-3.46, "Y"=0.0010030213007342376}, {"X"=-3.45, "Y"=0.0010382812956614103}, {"X"=-3.44, "Y"=0.0010746733401537356}, {"X"=-3.43, "Y"=0.0011122297072655649}, {"X"=-3.42, "Y"=0.0011509834441784845}, {"X"=-3.41, "Y"=0.0011909683858061168}, {"X"=-3.4, "Y"=0.00123221916847302}, {"X"=-3.39, "Y"=0.001274771243661833}, {"X"=-3.38, "Y"=0.0013186608918227423}, {"X"=-3.37, "Y"=0.0013639252362389036}, {"X"=-3.36, "Y"=0.001410602256941385}, {"X"=-3.35, "Y"=0.0014587308046667459}, {"X"=-3.34, "Y"=0.0015083506148503075}, {"X"=-3.33, "Y"=0.0015595023216476915}, {"X"=-3.32, "Y"=0.0016122274719771244}, {"X"=-3.31, "Y"=0.0016665685395745797}, {"X"=-3.3, "Y"=0.0017225689390536812}, {"X"=-3.29, "Y"=0.0017802730399618788}, {"X"=-3.28, "Y"=0.0018397261808242812}, {"X"=-3.27, "Y"=0.0019009746831660803}, {"X"=-3.26, "Y"=0.001964065865504376}, {"X"=-3.25, "Y"=0.002029048057299768}, {"X"=-3.24, "Y"=0.002095970612857942}, {"X"=-3.23, "Y"=0.0021648839251710624}, {"X"=-3.22, "Y"=0.0022358394396885385}, {"X"=-3.21, "Y"=0.0023088896680064958}, {"X"=-3.2, "Y"=0.0023840882014648404}, {"X"=-3.19, "Y"=0.0024614897246407006}, {"X"=-3.18, "Y"=0.002541150028726522}, {"X"=-3.17, "Y"=0.0026231260247810244}, {"X"=-3.16, "Y"=0.0027074757568407003}, {"X"=-3.15, "Y"=0.002794258414879447}, {"X"=-3.14, "Y"=0.002883534347603439}, {"X"=-3.13, "Y"=0.002975365075068254}, {"X"=-3.12, "Y"=0.0030698133011047403}, {"X"=-3.11, "Y"=0.0031669429255400815}, {"X"=-3.1, "Y"=0.0032668190561999186}, {"X"=-3.09, "Y"=0.0033695080206774812}, {"X"=-3.08, "Y"=0.003475077377854938}, {"X"=-3.07, "Y"=0.0035835959291623614}, {"X"=-3.06, "Y"=0.003695133729559035}, {"X"=-3.05, "Y"=0.0038097620982218104}, {"X"=-3.04, "Y"=0.003927553628924779}, {"X"=-3.03, "Y"=0.00404858220009443}, {"X"=-3.02, "Y"=0.004172922984523962}, {"X"=-3.01, "Y"=0.00430065245873045}, {"X"=-3.0, "Y"=0.0044318484119380075}, {"X"=-2.99, "Y"=0.004566589954670145}, {"X"=-2.98, "Y"=0.004704957526933979}, {"X"=-2.97, "Y"=0.004847032905978945}, {"X"=-2.96, "Y"=0.004992899213612376}, {"X"=-2.95, "Y"=0.005142640923053939}, {"X"=-2.94, "Y"=0.00529634386531102}, {"X"=-2.93, "Y"=0.005454095235056545}, {"X"=-2.92, "Y"=0.005615983595990969}, {"X"=-2.91, "Y"=0.005782098885669473}, {"X"=-2.9, "Y"=0.005952532419775854}, {"X"=-2.89, "Y"=0.006127376895823688}, {"X"=-2.88, "Y"=0.0063067263962659275}, {"X"=-2.87, "Y"=0.006490676390993364}, {"X"=-2.86, "Y"=0.00667932373920262}, {"X"=-2.85, "Y"=0.006872766690613971}, {"X"=-2.84, "Y"=0.007071104886019449}, {"X"=-2.83, "Y"=0.007274439357141218}, {"X"=-2.82, "Y"=0.007482872525780564}, {"X"=-2.81, "Y"=0.007696508202237322}, {"X"=-2.8, "Y"=0.007915451582979969}, {"X"=-2.79, "Y"=0.008139809247546021}, {"X"=-2.78, "Y"=0.008369689154653033}, {"X"=-2.77, "Y"=0.008605200637499673}, {"X"=-2.76, "Y"=0.008846454398237232}, {"X"=-2.75, "Y"=0.009093562501591053}, {"X"=-2.74, "Y"=0.009346638367612283}, {"X"=-2.73, "Y"=0.009605796763539587}, {"X"=-2.72, "Y"=0.009871153794751132}, {"X"=-2.71, "Y"=0.010142826894787078}, {"X"=-2.7, "Y"=0.010420934814422592}, {"X"=-2.69, "Y"=0.010705597609772188}, {"X"=-2.68, "Y"=0.010996936629405572}, {"X"=-2.67, "Y"=0.011295074500456135}, {"X"=-2.66, "Y"=0.011600135113702562}, {"X"=-2.65, "Y"=0.01191224360760518}, {"X"=-2.64, "Y"=0.012231526351277971}, {"X"=-2.63, "Y"=0.012558110926378211}, {"X"=-2.62, "Y"=0.012892126107895304}, {"X"=-2.61, "Y"=0.013233701843821374}, {"X"=-2.6, "Y"=0.013582969233685615}, {"X"=-2.59, "Y"=0.013940060505935825}, {"X"=-2.58, "Y"=0.014305108994149692}, {"X"=-2.57, "Y"=0.014678249112060044}, {"X"=-2.56, "Y"=0.01505961632737745}, {"X"=-2.55, "Y"=0.015449347134395174}, {"X"=-2.54, "Y"=0.015847579025360818}, {"X"=-2.53, "Y"=0.016254450460600506}, {"X"=-2.52, "Y"=0.016670100837381057}, {"X"=-2.51, "Y"=0.017094670457496956}, {"X"=-2.5, "Y"=0.01752830049356854}, {"X"=-2.49, "Y"=0.017971132954039633}, {"X"=-2.48, "Y"=0.01842331064686205}, {"X"=-2.47, "Y"=0.018884977141856163}, {"X"=-2.46, "Y"=0.019356276731736965}, {"X"=-2.45, "Y"=0.019837354391795313}, {"X"=-2.44, "Y"=0.02032835573822584}, {"X"=-2.43, "Y"=0.020829426985092186}, {"X"=-2.42, "Y"=0.021340714899922786}, {"X"=-2.41, "Y"=0.021862366757929387}, {"X"=-2.4, "Y"=0.0223945302948429}, {"X"=-2.39, "Y"=0.022937353658360693}, {"X"=-2.38, "Y"=0.023490985358201367}, {"X"=-2.37, "Y"=0.02405557421476297}, {"X"=-2.36, "Y"=0.024631269306382507}, {"X"=-2.35, "Y"=0.025218219915194382}, {"X"=-2.34, "Y"=0.02581657547158769}, {"X"=-2.33, "Y"=0.026426485497261724}, {"X"=-2.32, "Y"=0.027048099546881785}, {"X"=-2.31, "Y"=0.027681567148336573}, {"X"=-2.3, "Y"=0.02832703774160119}, {"X"=-2.29, "Y"=0.028984660616209416}, {"X"=-2.28, "Y"=0.029654584847341278}, {"X"=-2.27, "Y"=0.03033695923053164}, {"X"=-2.26, "Y"=0.031031932215008273}, {"X"=-2.25, "Y"=0.03173965183566742}, {"X"=-2.24, "Y"=0.032460265643697445}, {"X"=-2.23, "Y"=0.03319392063586112}, {"X"=-2.22, "Y"=0.033940763182449186}, {"X"=-2.21, "Y"=0.03470093895391882}, {"X"=-2.2, "Y"=0.035474592846231424}, {"X"=-2.19, "Y"=0.03626186890490622}, {"X"=-2.18, "Y"=0.037062910247806474}, {"X"=-2.17, "Y"=0.03787785898667748}, {"X"=-2.16, "Y"=0.03870685614745561}, {"X"=-2.15, "Y"=0.03955004158937022}, {"X"=-2.14, "Y"=0.04040755392286031}, {"X"=-2.13, "Y"=0.041279530426330424}, {"X"=-2.12, "Y"=0.04216610696177031}, {"X"=-2.11, "Y"=0.04306741788926574}, {"X"=-2.1, "Y"=0.0439835959804272}, {"X"=-2.09, "Y"=0.0449147723307671}, {"X"=-2.08, "Y"=0.045861076271054894}, {"X"=-2.07, "Y"=0.04682263527768316}, {"X"=-2.06, "Y"=0.047799574882077034}, {"X"=-2.05, "Y"=0.04879201857918277}, {"X"=-2.04, "Y"=0.049800087735070775}, {"X"=-2.03, "Y"=0.05082390149369121}, {"X"=-2.02, "Y"=0.051863576682820565}, {"X"=-2.01, "Y"=0.05291922771924032}, {"X"=-2.0, "Y"=0.05399096651318806}, {"X"=-1.99, "Y"=0.05507890237212577}, {"X"=-1.98, "Y"=0.05618314190386805}, {"X"=-1.97, "Y"=0.05730378891911713}, {"X"=-1.96, "Y"=0.058440944333451476}, {"X"=-1.95, "Y"=0.059594706068816075}, {"X"=-1.94, "Y"=0.06076516895456478}, {"X"=-1.93, "Y"=0.061952424628105164}, {"X"=-1.92, "Y"=0.06315656143519865}, {"X"=-1.91, "Y"=0.06437766432996936}, {"X"=-1.9, "Y"=0.0656158147746766}, {"X"=-1.89, "Y"=0.06687109063930716}, {"X"=-1.88, "Y"=0.06814356610104459}, {"X"=-1.87, "Y"=0.06943331154367419}, {"X"=-1.86, "Y"=0.07074039345698338}, {"X"=-1.85, "Y"=0.072064874336218}, {"X"=-1.84, "Y"=0.07340681258165689}, {"X"=-1.83, "Y"=0.0747662623983676}, {"X"=-1.82, "Y"=0.07614327369620731}, {"X"=-1.81, "Y"=0.07753789199013399}, {"X"=-1.8, "Y"=0.07895015830089415}, {"X"=-1.79, "Y"=0.08038010905615417}, {"X"=-1.78, "Y"=0.08182777599214282}, {"X"=-1.77, "Y"=0.08329318605587446}, {"X"=-1.76, "Y"=0.08477636130802224}, {"X"=-1.75, "Y"=0.08627731882651153}, {"X"=-1.74, "Y"=0.08779607061090564}, {"X"=-1.73, "Y"=0.089332623487655}, {"X"=-1.72, "Y"=0.09088697901628288}, {"X"=-1.71, "Y"=0.09245913339658068}, {"X"=-1.7, "Y"=0.09404907737688695}, {"X"=-1.69, "Y"=0.09565679616352402}, {"X"=-1.68, "Y"=0.09728226933146752}, {"X"=-1.67, "Y"=0.09892547073632373}, {"X"=-1.66, "Y"=0.10058636842769057}, {"X"=-1.65, "Y"=0.10226492456397804}, {"X"=-1.64, "Y"=0.10396109532876424}, {"X"=-1.63, "Y"=0.10567483084876363}, {"X"=-1.62, "Y"=0.1074060751134838}, {"X"=-1.61, "Y"=0.10915476589664735}, {"X"=-1.6, "Y"=0.11092083467945554}, {"X"=-1.59, "Y"=0.11270420657577056}, {"X"=-1.58, "Y"=0.11450480025929236}, {"X"=-1.57, "Y"=0.1163225278928071}, {"X"=-1.56, "Y"=0.11815729505958228}, {"X"=-1.55, "Y"=0.12000900069698558}, {"X"=-1.54, "Y"=0.12187753703240178}, {"X"=-1.53, "Y"=0.12376278952152314}, {"X"=-1.52, "Y"=0.12566463678908815}, {"X"=-1.51, "Y"=0.12758295057214186}, {"X"=-1.5, "Y"=0.12951759566589174}, {"X"=-1.49, "Y"=0.13146842987223106}, {"X"=-1.48, "Y"=0.13343530395100234}, {"X"=-1.47, "Y"=0.1354180615740713}, {"X"=-1.46, "Y"=0.13741653928228179}, {"X"=-1.45, "Y"=0.13943056644536028}, {"X"=-1.44, "Y"=0.1414599652248388}, {"X"=-1.43, "Y"=0.14350455054006242}, {"X"=-1.42, "Y"=0.1455641300373476}, {"X"=-1.41, "Y"=0.14763850406235574}, {"X"=-1.4, "Y"=0.14972746563574488}, {"X"=-1.39, "Y"=0.1518308004321617}, {"X"=-1.38, "Y"=0.15394828676263372}, {"X"=-1.37, "Y"=0.15607969556042084}, {"X"=-1.36, "Y"=0.15822479037038303}, {"X"=-1.35, "Y"=0.1603833273419196}, {"X"=-1.34, "Y"=0.16255505522553412}, {"X"=-1.33, "Y"=0.1647397153730768}, {"X"=-1.32, "Y"=0.1669370417417138}, {"X"=-1.31, "Y"=0.1691467609016724}, {"X"=-1.3, "Y"=0.17136859204780736}, {"X"=-1.29, "Y"=0.173602247015033}, {"X"=-1.28, "Y"=0.17584743029766237}, {"X"=-1.27, "Y"=0.1781038390726936}, {"X"=-1.26, "Y"=0.18037116322708033}, {"X"=-1.25, "Y"=0.18264908538902191}, {"X"=-1.24, "Y"=0.1849372809633053}, {"X"=-1.23, "Y"=0.18723541817072956}, {"X"=-1.22, "Y"=0.18954315809164027}, {"X"=-1.21, "Y"=0.1918601547135994}, {"X"=-1.2, "Y"=0.19418605498321298}, {"X"=-1.19, "Y"=0.19652049886213654}, {"X"=-1.18, "Y"=0.1988631193872759}, {"X"=-1.17, "Y"=0.2012135427351974}, {"X"=-1.16, "Y"=0.20357138829075944}, {"X"=-1.15, "Y"=0.20593626871997478}, {"X"=-1.14, "Y"=0.20830779004710837}, {"X"=-1.13, "Y"=0.21068555173601533}, {"X"=-1.12, "Y"=0.21306914677571784}, {"X"=-1.11, "Y"=0.2154581617702197}, {"X"=-1.1, "Y"=0.21785217703255055}, {"X"=-1.09, "Y"=0.22025076668303326}, {"X"=-1.08, "Y"=0.22265349875176116}, {"X"=-1.07, "Y"=0.22505993528526969}, {"X"=-1.06, "Y"=0.2274696324573859}, {"X"=-1.05, "Y"=0.22988214068423302}, {"X"=-1.04, "Y"=0.2322970047433662}, {"X"=-1.03, "Y"=0.23471376389701185}, {"X"=-1.02, "Y"=0.23713195201937962}, {"X"=-1.01, "Y"=0.23955109772801336}, {"X"=-1.0, "Y"=0.24197072451914337}, {"X"=-0.99, "Y"=0.2443903509069996}, {"X"=-0.98, "Y"=0.24680949056704274}, {"X"=-0.97, "Y"=0.24922765248306594}, {"X"=-0.96, "Y"=0.2516443410981171}, {"X"=-0.95, "Y"=0.254059056469189}, {"X"=-0.94, "Y"=0.25647129442562033}, {"X"=-0.93, "Y"=0.25888054673114885}, {"X"=-0.92, "Y"=0.26128630124955315}, {"X"=-0.91, "Y"=0.2636880421138182}, {"X"=-0.9, "Y"=0.2660852498987548}, {"X"=-0.89, "Y"=0.2684774017970024}, {"X"=-0.88, "Y"=0.27086397179833804}, {"X"=-0.87, "Y"=0.2732444308722162}, {"X"=-0.86, "Y"=0.27561824715345673}, {"X"=-0.85, "Y"=0.2779848861309965}, {"X"=-0.84, "Y"=0.2803438108396206}, {"X"=-0.83, "Y"=0.28269448205458025}, {"X"=-0.82, "Y"=0.28503635848900727}, {"X"=-0.81, "Y"=0.2873688969940283}, {"X"=-0.8, "Y"=0.28969155276148273}, {"X"=-0.79, "Y"=0.2920037795291414}, {"X"=-0.78, "Y"=0.2943050297883251}, {"X"=-0.77, "Y"=0.2965947549938157}, {"X"=-0.76, "Y"=0.29887240577595275}, {"X"=-0.75, "Y"=0.30113743215480443}, {"X"=-0.74, "Y"=0.30338928375630014}, {"X"=-0.73, "Y"=0.30562741003020993}, {"X"=-0.72, "Y"=0.30785126046985295}, {"X"=-0.71, "Y"=0.31006028483341613}, {"X"=-0.7, "Y"=0.31225393336676127}, {"X"=-0.69, "Y"=0.31443165702759734}, {"X"=-0.68, "Y"=0.31659290771089277}, {"X"=-0.67, "Y"=0.3187371384754015}, {"X"=-0.66, "Y"=0.3208638037711725}, {"X"=-0.65, "Y"=0.3229723596679143}, {"X"=-0.64, "Y"=0.3250622640840822}, {"X"=-0.63, "Y"=0.3271329770165545}, {"X"=-0.62, "Y"=0.3291839607707648}, {"X"=-0.61, "Y"=0.33121468019115297}, {"X"=-0.6, "Y"=0.33322460289179967}, {"X"=-0.59, "Y"=0.33521319948710615}, {"X"=-0.58, "Y"=0.3371799438223806}, {"X"=-0.57, "Y"=0.33912431320419223}, {"X"=-0.56, "Y"=0.34104578863035256}, {"X"=-0.55, "Y"=0.3429438550193839}, {"X"=-0.54, "Y"=0.3448180014393334}, {"X"=-0.53, "Y"=0.34666772133579166}, {"X"=-0.52, "Y"=0.3484925127589745}, {"X"=-0.51, "Y"=0.3502918785897258}, {"X"=-0.5, "Y"=0.3520653267642995}, {"X"=-0.49, "Y"=0.3538123704977797}, {"X"=-0.48, "Y"=0.3555325285059971}, {"X"=-0.47, "Y"=0.35722532522580086}, {"X"=-0.46, "Y"=0.35889029103354464}, {"X"=-0.45, "Y"=0.36052696246164795}, {"X"=-0.44, "Y"=0.3621348824130922}, {"X"=-0.43, "Y"=0.3637136003737134}, {"X"=-0.42, "Y"=0.3652626726221539}, {"X"=-0.41, "Y"=0.3667816624373361}, {"X"=-0.4, "Y"=0.36827014030332333}, {"X"=-0.39, "Y"=0.36972768411143236}, {"X"=-0.38, "Y"=0.37115387935946603}, {"X"=-0.37, "Y"=0.3725483193479334}, {"X"=-0.36, "Y"=0.3739106053731284}, {"X"=-0.35, "Y"=0.3752403469169379}, {"X"=-0.34, "Y"=0.376537161833254}, {"X"=-0.33, "Y"=0.37780067653086463}, {"X"=-0.32, "Y"=0.3790305261527017}, {"X"=-0.31, "Y"=0.38022635475132494}, {"X"=-0.3, "Y"=0.38138781546052414}, {"X"=-0.29, "Y"=0.38251457066292405}, {"X"=-0.28, "Y"=0.3836062921534786}, {"X"=-0.27, "Y"=0.3846626612987428}, {"X"=-0.26, "Y"=0.3856833691918161}, {"X"=-0.25, "Y"=0.3866681168028493}, {"X"=-0.24, "Y"=0.38761661512501416}, {"X"=-0.23, "Y"=0.3885285853158359}, {"X"=-0.22, "Y"=0.38940375883379047}, {"X"=-0.21, "Y"=0.39024187757007434}, {"X"=-0.2, "Y"=0.3910426939754559}, {"X"=-0.19, "Y"=0.3918059711821211}, {"X"=-0.18, "Y"=0.3925314831204289}, {"X"=-0.17, "Y"=0.3932190146304972}, {"X"=-0.16, "Y"=0.3938683615685408}, {"X"=-0.15, "Y"=0.39447933090788895}, {"X"=-0.14, "Y"=0.39505174083461125}, {"X"=-0.13, "Y"=0.3955854208376874}, {"X"=-0.12, "Y"=0.3960802117936561}, {"X"=-0.11, "Y"=0.3965359660456858}, {"X"=-0.1, "Y"=0.3969525474770118}, {"X"=-0.09, "Y"=0.39732983157868834}, {"X"=-0.08, "Y"=0.3976677055116089}, {"X"=-0.07, "Y"=0.39796606816275104}, {"X"=-0.06, "Y"=0.39822483019560695}, {"X"=-0.05, "Y"=0.39844391409476404}, {"X"=-0.04, "Y"=0.39862325420460504}, {"X"=-0.03, "Y"=0.39876279676209975}, {"X"=-0.02, "Y"=0.3988624999236661}, {"X"=-0.01, "Y"=0.39892233378608216}, {"X"=0.0, "Y"=0.3989422804014327}, {"X"=-0.0, "Y"=0.3989422804014327}, {"X"=0.01, "Y"=0.39892233378608216}, {"X"=0.02, "Y"=0.3988624999236661}, {"X"=0.03, "Y"=0.39876279676209975}, {"X"=0.04, "Y"=0.39862325420460504}, {"X"=0.05, "Y"=0.39844391409476404}, {"X"=0.06, "Y"=0.39822483019560695}, {"X"=0.07, "Y"=0.39796606816275104}, {"X"=0.08, "Y"=0.3976677055116089}, {"X"=0.09, "Y"=0.39732983157868834}, {"X"=0.1, "Y"=0.3969525474770118}, {"X"=0.11, "Y"=0.3965359660456858}, {"X"=0.12, "Y"=0.3960802117936561}, {"X"=0.13, "Y"=0.3955854208376874}, {"X"=0.14, "Y"=0.39505174083461125}, {"X"=0.15, "Y"=0.39447933090788895}, {"X"=0.16, "Y"=0.3938683615685408}, {"X"=0.17, "Y"=0.3932190146304972}, {"X"=0.18, "Y"=0.3925314831204289}, {"X"=0.19, "Y"=0.3918059711821211}, {"X"=0.2, "Y"=0.3910426939754559}, {"X"=0.21, "Y"=0.39024187757007434}, {"X"=0.22, "Y"=0.38940375883379047}, {"X"=0.23, "Y"=0.3885285853158359}, {"X"=0.24, "Y"=0.38761661512501416}, {"X"=0.25, "Y"=0.3866681168028493}, {"X"=0.26, "Y"=0.3856833691918161}, {"X"=0.27, "Y"=0.3846626612987428}, {"X"=0.28, "Y"=0.3836062921534786}, {"X"=0.29, "Y"=0.38251457066292405}, {"X"=0.3, "Y"=0.38138781546052414}, {"X"=0.31, "Y"=0.38022635475132494}, {"X"=0.32, "Y"=0.3790305261527017}, {"X"=0.33, "Y"=0.37780067653086463}, {"X"=0.34, "Y"=0.376537161833254}, {"X"=0.35, "Y"=0.3752403469169379}, {"X"=0.36, "Y"=0.3739106053731284}, {"X"=0.37, "Y"=0.3725483193479334}, {"X"=0.38, "Y"=0.37115387935946603}, {"X"=0.39, "Y"=0.36972768411143236}, {"X"=0.4, "Y"=0.36827014030332333}, {"X"=0.41, "Y"=0.3667816624373361}, {"X"=0.42, "Y"=0.3652626726221539}, {"X"=0.43, "Y"=0.3637136003737134}, {"X"=0.44, "Y"=0.3621348824130922}, {"X"=0.45, "Y"=0.36052696246164795}, {"X"=0.46, "Y"=0.35889029103354464}, {"X"=0.47, "Y"=0.35722532522580086}, {"X"=0.48, "Y"=0.3555325285059971}, {"X"=0.49, "Y"=0.3538123704977797}, {"X"=0.5, "Y"=0.3520653267642995}, {"X"=0.51, "Y"=0.3502918785897258}, {"X"=0.52, "Y"=0.3484925127589745}, {"X"=0.53, "Y"=0.34666772133579166}, {"X"=0.54, "Y"=0.3448180014393334}, {"X"=0.55, "Y"=0.3429438550193839}, {"X"=0.56, "Y"=0.34104578863035256}, {"X"=0.57, "Y"=0.33912431320419223}, {"X"=0.58, "Y"=0.3371799438223806}, {"X"=0.59, "Y"=0.33521319948710615}, {"X"=0.6, "Y"=0.33322460289179967}, {"X"=0.61, "Y"=0.33121468019115297}, {"X"=0.62, "Y"=0.3291839607707648}, {"X"=0.63, "Y"=0.3271329770165545}, {"X"=0.64, "Y"=0.3250622640840822}, {"X"=0.65, "Y"=0.3229723596679143}, {"X"=0.66, "Y"=0.3208638037711725}, {"X"=0.67, "Y"=0.3187371384754015}, {"X"=0.68, "Y"=0.31659290771089277}, {"X"=0.69, "Y"=0.31443165702759734}, {"X"=0.7, "Y"=0.31225393336676127}, {"X"=0.71, "Y"=0.31006028483341613}, {"X"=0.72, "Y"=0.30785126046985295}, {"X"=0.73, "Y"=0.30562741003020993}, {"X"=0.74, "Y"=0.30338928375630014}, {"X"=0.75, "Y"=0.30113743215480443}, {"X"=0.76, "Y"=0.29887240577595275}, {"X"=0.77, "Y"=0.2965947549938157}, {"X"=0.78, "Y"=0.2943050297883251}, {"X"=0.79, "Y"=0.2920037795291414}, {"X"=0.8, "Y"=0.28969155276148273}, {"X"=0.81, "Y"=0.2873688969940283}, {"X"=0.82, "Y"=0.28503635848900727}, {"X"=0.83, "Y"=0.28269448205458025}, {"X"=0.84, "Y"=0.2803438108396206}, {"X"=0.85, "Y"=0.2779848861309965}, {"X"=0.86, "Y"=0.27561824715345673}, {"X"=0.87, "Y"=0.2732444308722162}, {"X"=0.88, "Y"=0.27086397179833804}, {"X"=0.89, "Y"=0.2684774017970024}, {"X"=0.9, "Y"=0.2660852498987548}, {"X"=0.91, "Y"=0.2636880421138182}, {"X"=0.92, "Y"=0.26128630124955315}, {"X"=0.93, "Y"=0.25888054673114885}, {"X"=0.94, "Y"=0.25647129442562033}, {"X"=0.95, "Y"=0.254059056469189}, {"X"=0.96, "Y"=0.2516443410981171}, {"X"=0.97, "Y"=0.24922765248306594}, {"X"=0.98, "Y"=0.24680949056704274}, {"X"=0.99, "Y"=0.2443903509069996}, {"X"=1.0, "Y"=0.24197072451914337}, {"X"=1.01, "Y"=0.23955109772801336}, {"X"=1.02, "Y"=0.23713195201937962}, {"X"=1.03, "Y"=0.23471376389701185}, {"X"=1.04, "Y"=0.2322970047433662}, {"X"=1.05, "Y"=0.22988214068423302}, {"X"=1.06, "Y"=0.2274696324573859}, {"X"=1.07, "Y"=0.22505993528526969}, {"X"=1.08, "Y"=0.22265349875176116}, {"X"=1.09, "Y"=0.22025076668303326}, {"X"=1.1, "Y"=0.21785217703255055}, {"X"=1.11, "Y"=0.2154581617702197}, {"X"=1.12, "Y"=0.21306914677571784}, {"X"=1.13, "Y"=0.21068555173601533}, {"X"=1.14, "Y"=0.20830779004710837}, {"X"=1.15, "Y"=0.20593626871997478}, {"X"=1.16, "Y"=0.20357138829075944}, {"X"=1.17, "Y"=0.2012135427351974}, {"X"=1.18, "Y"=0.1988631193872759}, {"X"=1.19, "Y"=0.19652049886213654}, {"X"=1.2, "Y"=0.19418605498321298}, {"X"=1.21, "Y"=0.1918601547135994}, {"X"=1.22, "Y"=0.18954315809164027}, {"X"=1.23, "Y"=0.18723541817072956}, {"X"=1.24, "Y"=0.1849372809633053}, {"X"=1.25, "Y"=0.18264908538902191}, {"X"=1.26, "Y"=0.18037116322708033}, {"X"=1.27, "Y"=0.1781038390726936}, {"X"=1.28, "Y"=0.17584743029766237}, {"X"=1.29, "Y"=0.173602247015033}, {"X"=1.3, "Y"=0.17136859204780736}, {"X"=1.31, "Y"=0.1691467609016724}, {"X"=1.32, "Y"=0.1669370417417138}, {"X"=1.33, "Y"=0.1647397153730768}, {"X"=1.34, "Y"=0.16255505522553412}, {"X"=1.35, "Y"=0.1603833273419196}, {"X"=1.36, "Y"=0.15822479037038303}, {"X"=1.37, "Y"=0.15607969556042084}, {"X"=1.38, "Y"=0.15394828676263372}, {"X"=1.39, "Y"=0.1518308004321617}, {"X"=1.4, "Y"=0.14972746563574488}, {"X"=1.41, "Y"=0.14763850406235574}, {"X"=1.42, "Y"=0.1455641300373476}, {"X"=1.43, "Y"=0.14350455054006242}, {"X"=1.44, "Y"=0.1414599652248388}, {"X"=1.45, "Y"=0.13943056644536028}, {"X"=1.46, "Y"=0.13741653928228179}, {"X"=1.47, "Y"=0.1354180615740713}, {"X"=1.48, "Y"=0.13343530395100234}, {"X"=1.49, "Y"=0.13146842987223106}, {"X"=1.5, "Y"=0.12951759566589174}, {"X"=1.51, "Y"=0.12758295057214186}, {"X"=1.52, "Y"=0.12566463678908815}, {"X"=1.53, "Y"=0.12376278952152314}, {"X"=1.54, "Y"=0.12187753703240178}, {"X"=1.55, "Y"=0.12000900069698558}, {"X"=1.56, "Y"=0.11815729505958228}, {"X"=1.57, "Y"=0.1163225278928071}, {"X"=1.58, "Y"=0.11450480025929236}, {"X"=1.59, "Y"=0.11270420657577056}, {"X"=1.6, "Y"=0.11092083467945554}, {"X"=1.61, "Y"=0.10915476589664735}, {"X"=1.62, "Y"=0.1074060751134838}, {"X"=1.63, "Y"=0.10567483084876363}, {"X"=1.64, "Y"=0.10396109532876424}, {"X"=1.65, "Y"=0.10226492456397804}, {"X"=1.66, "Y"=0.10058636842769057}, {"X"=1.67, "Y"=0.09892547073632373}, {"X"=1.68, "Y"=0.09728226933146752}, {"X"=1.69, "Y"=0.09565679616352402}, {"X"=1.7, "Y"=0.09404907737688695}, {"X"=1.71, "Y"=0.09245913339658068}, {"X"=1.72, "Y"=0.09088697901628288}, {"X"=1.73, "Y"=0.089332623487655}, {"X"=1.74, "Y"=0.08779607061090564}, {"X"=1.75, "Y"=0.08627731882651153}, {"X"=1.76, "Y"=0.08477636130802224}, {"X"=1.77, "Y"=0.08329318605587446}, {"X"=1.78, "Y"=0.08182777599214282}, {"X"=1.79, "Y"=0.08038010905615417}, {"X"=1.8, "Y"=0.07895015830089415}, {"X"=1.81, "Y"=0.07753789199013399}, {"X"=1.82, "Y"=0.07614327369620731}, {"X"=1.83, "Y"=0.0747662623983676}, {"X"=1.84, "Y"=0.07340681258165689}, {"X"=1.85, "Y"=0.072064874336218}, {"X"=1.86, "Y"=0.07074039345698338}, {"X"=1.87, "Y"=0.06943331154367419}, {"X"=1.88, "Y"=0.06814356610104459}, {"X"=1.89, "Y"=0.06687109063930716}, {"X"=1.9, "Y"=0.0656158147746766}, {"X"=1.91, "Y"=0.06437766432996936}, {"X"=1.92, "Y"=0.06315656143519865}, {"X"=1.93, "Y"=0.061952424628105164}, {"X"=1.94, "Y"=0.06076516895456478}, {"X"=1.95, "Y"=0.059594706068816075}, {"X"=1.96, "Y"=0.058440944333451476}, {"X"=1.97, "Y"=0.05730378891911713}, {"X"=1.98, "Y"=0.05618314190386805}, {"X"=1.99, "Y"=0.05507890237212577}, {"X"=2.0, "Y"=0.05399096651318806}, {"X"=2.01, "Y"=0.05291922771924032}, {"X"=2.02, "Y"=0.051863576682820565}, {"X"=2.03, "Y"=0.05082390149369121}, {"X"=2.04, "Y"=0.049800087735070775}, {"X"=2.05, "Y"=0.04879201857918277}, {"X"=2.06, "Y"=0.047799574882077034}, {"X"=2.07, "Y"=0.04682263527768316}, {"X"=2.08, "Y"=0.045861076271054894}, {"X"=2.09, "Y"=0.0449147723307671}, {"X"=2.1, "Y"=0.0439835959804272}, {"X"=2.11, "Y"=0.04306741788926574}, {"X"=2.12, "Y"=0.04216610696177031}, {"X"=2.13, "Y"=0.041279530426330424}, {"X"=2.14, "Y"=0.04040755392286031}, {"X"=2.15, "Y"=0.03955004158937022}, {"X"=2.16, "Y"=0.03870685614745561}, {"X"=2.17, "Y"=0.03787785898667748}, {"X"=2.18, "Y"=0.037062910247806474}, {"X"=2.19, "Y"=0.03626186890490622}, {"X"=2.2, "Y"=0.035474592846231424}, {"X"=2.21, "Y"=0.03470093895391882}, {"X"=2.22, "Y"=0.033940763182449186}, {"X"=2.23, "Y"=0.03319392063586112}, {"X"=2.24, "Y"=0.032460265643697445}, {"X"=2.25, "Y"=0.03173965183566742}, {"X"=2.26, "Y"=0.031031932215008273}, {"X"=2.27, "Y"=0.03033695923053164}, {"X"=2.28, "Y"=0.029654584847341278}, {"X"=2.29, "Y"=0.028984660616209416}, {"X"=2.3, "Y"=0.02832703774160119}, {"X"=2.31, "Y"=0.027681567148336573}, {"X"=2.32, "Y"=0.027048099546881785}, {"X"=2.33, "Y"=0.026426485497261724}, {"X"=2.34, "Y"=0.02581657547158769}, {"X"=2.35, "Y"=0.025218219915194382}, {"X"=2.36, "Y"=0.024631269306382507}, {"X"=2.37, "Y"=0.02405557421476297}, {"X"=2.38, "Y"=0.023490985358201367}, {"X"=2.39, "Y"=0.022937353658360693}, {"X"=2.4, "Y"=0.0223945302948429}, {"X"=2.41, "Y"=0.021862366757929387}, {"X"=2.42, "Y"=0.021340714899922786}, {"X"=2.43, "Y"=0.020829426985092186}, {"X"=2.44, "Y"=0.02032835573822584}, {"X"=2.45, "Y"=0.019837354391795313}, {"X"=2.46, "Y"=0.019356276731736965}, {"X"=2.47, "Y"=0.018884977141856163}, {"X"=2.48, "Y"=0.01842331064686205}, {"X"=2.49, "Y"=0.017971132954039633}, {"X"=2.5, "Y"=0.01752830049356854}, {"X"=2.51, "Y"=0.017094670457496956}, {"X"=2.52, "Y"=0.016670100837381057}, {"X"=2.53, "Y"=0.016254450460600506}, {"X"=2.54, "Y"=0.015847579025360818}, {"X"=2.55, "Y"=0.015449347134395174}, {"X"=2.56, "Y"=0.01505961632737745}, {"X"=2.57, "Y"=0.014678249112060044}, {"X"=2.58, "Y"=0.014305108994149692}, {"X"=2.59, "Y"=0.013940060505935825}, {"X"=2.6, "Y"=0.013582969233685615}, {"X"=2.61, "Y"=0.013233701843821374}, {"X"=2.62, "Y"=0.012892126107895304}, {"X"=2.63, "Y"=0.012558110926378211}, {"X"=2.64, "Y"=0.012231526351277971}, {"X"=2.65, "Y"=0.01191224360760518}, {"X"=2.66, "Y"=0.011600135113702562}, {"X"=2.67, "Y"=0.011295074500456135}, {"X"=2.68, "Y"=0.010996936629405572}, {"X"=2.69, "Y"=0.010705597609772188}, {"X"=2.7, "Y"=0.010420934814422592}, {"X"=2.71, "Y"=0.010142826894787078}, {"X"=2.72, "Y"=0.009871153794751132}, {"X"=2.73, "Y"=0.009605796763539587}, {"X"=2.74, "Y"=0.009346638367612283}, {"X"=2.75, "Y"=0.009093562501591053}, {"X"=2.76, "Y"=0.008846454398237232}, {"X"=2.77, "Y"=0.008605200637499673}, {"X"=2.78, "Y"=0.008369689154653033}, {"X"=2.79, "Y"=0.008139809247546021}, {"X"=2.8, "Y"=0.007915451582979969}, {"X"=2.81, "Y"=0.007696508202237322}, {"X"=2.82, "Y"=0.007482872525780564}, {"X"=2.83, "Y"=0.007274439357141218}, {"X"=2.84, "Y"=0.007071104886019449}, {"X"=2.85, "Y"=0.006872766690613971}, {"X"=2.86, "Y"=0.00667932373920262}, {"X"=2.87, "Y"=0.006490676390993364}, {"X"=2.88, "Y"=0.0063067263962659275}, {"X"=2.89, "Y"=0.006127376895823688}, {"X"=2.9, "Y"=0.005952532419775854}, {"X"=2.91, "Y"=0.005782098885669473}, {"X"=2.92, "Y"=0.005615983595990969}, {"X"=2.93, "Y"=0.005454095235056545}, {"X"=2.94, "Y"=0.00529634386531102}, {"X"=2.95, "Y"=0.005142640923053939}, {"X"=2.96, "Y"=0.004992899213612376}, {"X"=2.97, "Y"=0.004847032905978945}, {"X"=2.98, "Y"=0.004704957526933979}, {"X"=2.99, "Y"=0.004566589954670145}, {"X"=3.0, "Y"=0.0044318484119380075}, {"X"=3.01, "Y"=0.00430065245873045}, {"X"=3.02, "Y"=0.004172922984523962}, {"X"=3.03, "Y"=0.00404858220009443}, {"X"=3.04, "Y"=0.003927553628924779}, {"X"=3.05, "Y"=0.0038097620982218104}, {"X"=3.06, "Y"=0.003695133729559035}, {"X"=3.07, "Y"=0.0035835959291623614}, {"X"=3.08, "Y"=0.003475077377854938}, {"X"=3.09, "Y"=0.0033695080206774812}, {"X"=3.1, "Y"=0.0032668190561999186}, {"X"=3.11, "Y"=0.0031669429255400815}, {"X"=3.12, "Y"=0.0030698133011047403}, {"X"=3.13, "Y"=0.002975365075068254}, {"X"=3.14, "Y"=0.002883534347603439}, {"X"=3.15, "Y"=0.002794258414879447}, {"X"=3.16, "Y"=0.0027074757568407003}, {"X"=3.17, "Y"=0.0026231260247810244}, {"X"=3.18, "Y"=0.002541150028726522}, {"X"=3.19, "Y"=0.0024614897246407006}, {"X"=3.2, "Y"=0.0023840882014648404}, {"X"=3.21, "Y"=0.0023088896680064958}, {"X"=3.22, "Y"=0.0022358394396885385}, {"X"=3.23, "Y"=0.0021648839251710624}, {"X"=3.24, "Y"=0.002095970612857942}, {"X"=3.25, "Y"=0.002029048057299768}, {"X"=3.26, "Y"=0.001964065865504376}, {"X"=3.27, "Y"=0.0019009746831660803}, {"X"=3.28, "Y"=0.0018397261808242812}, {"X"=3.29, "Y"=0.0017802730399618788}, {"X"=3.3, "Y"=0.0017225689390536812}, {"X"=3.31, "Y"=0.0016665685395745797}, {"X"=3.32, "Y"=0.0016122274719771244}, {"X"=3.33, "Y"=0.0015595023216476915}, {"X"=3.34, "Y"=0.0015083506148503075}, {"X"=3.35, "Y"=0.0014587308046667459}, {"X"=3.36, "Y"=0.001410602256941385}, {"X"=3.37, "Y"=0.0013639252362389036}, {"X"=3.38, "Y"=0.0013186608918227423}, {"X"=3.39, "Y"=0.001274771243661833}, {"X"=3.4, "Y"=0.00123221916847302}, {"X"=3.41, "Y"=0.0011909683858061168}, {"X"=3.42, "Y"=0.0011509834441784845}, {"X"=3.43, "Y"=0.0011122297072655649}, {"X"=3.44, "Y"=0.0010746733401537356}, {"X"=3.45, "Y"=0.0010382812956614103}, {"X"=3.46, "Y"=0.0010030213007342376}, {"X"=3.47, "Y"=0.0009688618429198459}, {"X"=3.48, "Y"=0.0009357721569274798}, {"X"=3.49, "Y"=0.0009037222112775245}, {"X"=3.5, "Y"=0.0008726826950457602}, {"X"=3.51, "Y"=0.0008426250047069028}, {"X"=3.52, "Y"=0.0008135212310818085}, {"X"=3.53, "Y"=0.00078534414639247}, {"X"=3.54, "Y"=0.0007580671914287103}, {"X"=3.55, "Y"=0.0007316644628303109}, {"X"=3.56, "Y"=0.0007061107004880362}, {"X"=3.57, "Y"=0.0006813812750668921}, {"X"=3.58, "Y"=0.0006574521756546766}, {"X"=3.59, "Y"=0.0006342999975387576}, {"X"=3.6, "Y"=0.0006119019301137719}, {"X"=3.61, "Y"=0.0005902357449227856}, {"X"=3.62, "Y"=0.0005692797838342526}, {"X"=3.63, "Y"=0.0005490129473569587}, {"X"=3.64, "Y"=0.0005294146830949348}, {"X"=3.65, "Y"=0.0005104649743441856}, {"X"=3.66, "Y"=0.0004921443288328931}, {"X"=3.67, "Y"=0.00047443376760662064}, {"X"=3.68, "Y"=0.00045731481405985675}, {"X"=3.69, "Y"=0.0004407694831151325}, {"X"=3.7, "Y"=0.00042478027055075143}, {"X"=3.71, "Y"=0.0004093301424780789}, {"X"=3.72, "Y"=0.0003944025249691562}, {"X"=3.73, "Y"=0.00037998129383532146}, {"X"=3.74, "Y"=0.000366050764557335}, {"X"=3.75, "Y"=0.00035259568236744546}, {"X"=3.76, "Y"=0.0003396012124836548}, {"X"=3.77, "Y"=0.00032705293049637503}, {"X"=3.78, "Y"=0.0003149368129075219}, {"X"=3.79, "Y"=0.0003032392278220042}, {"X"=3.8, "Y"=0.00029194692579146027}, {"X"=3.81, "Y"=0.0002810470308099863}, {"X"=3.82, "Y"=0.000270527031461521}, {"X"=3.83, "Y"=0.00026037477221844247}, {"X"=3.84, "Y"=0.00025057844489086075}, {"X"=3.85, "Y"=0.00024112658022599324}, {"X"=3.86, "Y"=0.00023200803965694238}, {"X"=3.87, "Y"=0.0002232120072001021}, {"X"=3.88, "Y"=0.00021472798150036704}, {"X"=3.89, "Y"=0.00020654576802322548}, {"X"=3.9, "Y"=0.00019865547139277272}, {"X"=3.91, "Y"=0.00019104748787459762}, {"X"=3.92, "Y"=0.0001837124980024571}, {"X"=3.93, "Y"=0.00017664145934757092}, {"X"=3.94, "Y"=0.00016982559942934359}, {"X"=3.95, "Y"=0.00016325640876624202}, {"X"=3.96, "Y"=0.00015692563406553226}, {"X"=3.97, "Y"=0.0001508252715505178}, {"X"=3.98, "Y"=0.00014494756042389106}, {"X"=3.99, "Y"=0.00013928497646575994}, {"X"=4.0, "Y"=0.00013383022576488537}, {"X"=4.01, "Y"=0.00012857623858162108}, {"X"=4.02, "Y"=0.00012351616334102368}, {"X"=4.03, "Y"=0.00011864336075456578}, {"X"=4.04, "Y"=0.00011395139806886461}, {"X"=4.05, "Y"=0.00010943404343980055}, {"X"=4.06, "Y"=0.00010508526043040049}, {"X"=4.07, "Y"=0.00010089920263081443}, {"X"=4.08, "Y"=9.687020839871927e-05}, {"X"=4.09, "Y"=9.299279571844591e-05}, {"X"=4.1, "Y"=8.926165717713293e-05}, {"X"=4.11, "Y"=8.567165505618186e-05}, {"X"=4.12, "Y"=8.2217816536286e-05}, {"X"=4.13, "Y"=7.889532901429309e-05}, {"X"=4.14, "Y"=7.569953553016121e-05}, {"X"=4.15, "Y"=7.262593030225234e-05}, {"X"=4.16, "Y"=6.967015436921434e-05}, {"X"=4.17, "Y"=6.682799133669061e-05}, {"X"=4.18, "Y"=6.40953632271061e-05}, {"X"=4.19, "Y"=6.146832643076922e-05}, {"X"=4.2, "Y"=5.8943067756539855e-05}, {"X"=4.21, "Y"=5.651590058030741e-05}, {"X"=4.22, "Y"=5.4183261089540144e-05}, {"X"=4.23, "Y"=5.1941704622159776e-05}, {"X"=4.24, "Y"=4.978790209801209e-05}, {"X"=4.25, "Y"=4.771863654120495e-05}, {"X"=4.26, "Y"=4.5730799691601314e-05}, {"X"=4.27, "Y"=4.382138870375812e-05}, {"X"=4.28, "Y"=4.198750293161732e-05}, {"X"=4.29, "Y"=4.022634079726497e-05}, {"X"=4.3, "Y"=3.853519674208713e-05}, {"X"=4.31, "Y"=3.69114582586662e-05}, {"X"=4.32, "Y"=3.5352603001773097e-05}, {"X"=4.33, "Y"=3.385619597682789e-05}, {"X"=4.34, "Y"=3.241988680421378e-05}, {"X"=4.35, "Y"=3.1041407057850266e-05}, {"X"=4.36, "Y"=2.97185676764422e-05}, {"X"=4.37, "Y"=2.8449256445844308e-05}, {"X"=4.38, "Y"=2.723143555099261e-05}, {"X"=4.39, "Y"=2.6063139195878346e-05}, {"X"=4.4, "Y"=2.4942471290053535e-05}, {"X"=4.41, "Y"=2.38676032001796e-05}, {"X"=4.42, "Y"=2.283677156514692e-05}, {"X"=4.43, "Y"=2.184827617331647e-05}, {"X"=4.44, "Y"=2.0900477900450407e-05}, {"X"=4.45, "Y"=1.999179670692279e-05}, {"X"=4.46, "Y"=1.9120709692817737e-05}, {"X"=4.47, "Y"=1.828574920954738e-05}, {"X"=4.48, "Y"=1.748550102663914e-05}, {"X"=4.49, "Y"=1.671860255236507e-05}, {"X"=4.5, "Y"=1.5983741106905478e-05}, {"X"=4.51, "Y"=1.527965224676162e-05}, {"X"=4.52, "Y"=1.4605118139152942e-05}, {"X"=4.53, "Y"=1.3958965985154772e-05}, {"X"=4.54, "Y"=1.334006649035584e-05}, {"X"=4.55, "Y"=1.2747332381833467e-05}, {"X"=4.56, "Y"=1.21797169702687e-05}, {"X"=4.57, "Y"=1.1636212756042669e-05}, {"X"=4.58, "Y"=1.111585007817779e-05}, {"X"=4.59, "Y"=1.0617695805008393e-05}, {"X"=4.6, "Y"=1.014085206548676e-05}, {"X"=4.61, "Y"=9.684455020051437e-06}, {"X"=4.62, "Y"=9.247673670005617e-06}, {"X"=4.63, "Y"=8.829708704374098e-06}, {"X"=4.64, "Y"=8.429791383228772e-06}, {"X"=4.65, "Y"=8.047182456492295e-06}, {"X"=4.66, "Y"=7.681171117250455e-06}, {"X"=4.67, "Y"=7.331073988623946e-06}, {"X"=4.68, "Y"=6.996234143270405e-06}, {"X"=4.69, "Y"=6.676020154607462e-06}, {"X"=4.7, "Y"=6.36982517886709e-06}, {"X"=4.71, "Y"=6.077066067111116e-06}, {"X"=4.72, "Y"=5.797182506357288e-06}, {"X"=4.73, "Y"=5.529636188984052e-06}, {"X"=4.74, "Y"=5.273910009601304e-06}, {"X"=4.75, "Y"=5.029507288592446e-06}, {"X"=4.76, "Y"=4.795951021552522e-06}, {"X"=4.77, "Y"=4.5727831538641446e-06}, {"X"=4.78, "Y"=4.359563879671637e-06}, {"X"=4.79, "Y"=4.155870964531201e-06}, {"X"=4.8, "Y"=3.961299091032075e-06}, {"X"=4.81, "Y"=3.775459226701349e-06}, {"X"=4.82, "Y"=3.5979780135212474e-06}, {"X"=4.83, "Y"=3.428497178405039e-06}, {"X"=4.84, "Y"=3.266672963993275e-06}, {"X"=4.85, "Y"=3.112175579148945e-06}, {"X"=4.86, "Y"=2.964688668545273e-06}, {"X"=4.87, "Y"=2.823908800755821e-06}, {"X"=4.88, "Y"=2.6895449742715237e-06}, {"X"=4.89, "Y"=2.5613181408845447e-06}, {"X"=4.9, "Y"=2.438960745893352e-06}, {"X"=4.91, "Y"=2.322216284597997e-06}, {"X"=4.92, "Y"=2.2108388745684212e-06}, {"X"=4.93, "Y"=2.10459284318313e-06}, {"X"=4.94, "Y"=2.0032523299484894e-06}, {"X"=4.95, "Y"=1.906600903122811e-06}, {"X"=4.96, "Y"=1.8144311901820306e-06}, {"X"=4.97, "Y"=1.7265445216770736e-06}, {"X"=4.98, "Y"=1.6427505880450713e-06}, {"X"=4.99, "Y"=1.5628671089492902e-06}, {"X"=5.0, "Y"=1.4867195147342979e-06}, {"X"=5.01, "Y"=1.4141406395950037e-06}, {"X"=5.02, "Y"=1.3449704260694445e-06}, {"X"=5.03, "Y"=1.2790556404765742e-06}, {"X"=5.04, "Y"=1.216249598931318e-06}, {"X"=5.05, "Y"=1.1564119035797834e-06}, {"X"=5.06, "Y"=1.0994081887082052e-06}, {"X"=5.07, "Y"=1.0451098763893177e-06}, {"X"=5.08, "Y"=9.93393941339912e-07}, {"X"=5.09, "Y"=9.441426846730874e-07}, {"X"=5.1, "Y"=8.972435162383337e-07}, {"X"=5.11, "Y"=8.52588745251786e-07}, {"X"=5.12, "Y"=8.100753789281346e-07}, {"X"=5.13, "Y"=7.696049288345129e-07}, {"X"=5.14, "Y"=7.310832246953503e-07}, {"X"=5.15, "Y"=6.944202353855339e-07}, {"X"=5.16, "Y"=6.595298968575217e-07}, {"X"=5.17, "Y"=6.263299467558902e-07}, {"X"=5.18, "Y"=5.947417654807764e-07}, {"X"=5.19, "Y"=5.64690223469076e-07}, {"X"=5.2, "Y"=5.361035344697615e-07}, {"X"=5.21, "Y"=5.08913114596766e-07}, {"X"=5.22, "Y"=4.830534469499683e-07}, {"X"=5.23, "Y"=4.584619516015329e-07}, {"X"=5.24, "Y"=4.350788607515109e-07}, {"X"=5.25, "Y"=4.1284709886299984e-07}, {"X"=5.26, "Y"=3.9171216759348166e-07}, {"X"=5.27, "Y"=3.7162203534495063e-07}, {"X"=5.28, "Y"=3.525270312614038e-07}, {"X"=5.29, "Y"=3.3437974350798003e-07}, {"X"=5.3, "Y"=3.171349216715976e-07}, {"X"=5.31, "Y"=3.007493831283838e-07}, {"X"=5.32, "Y"=2.851819232283976e-07}, {"X"=5.33, "Y"=2.7039322915329305e-07}, {"X"=5.34, "Y"=2.5634579730745934e-07}, {"X"=5.35, "Y"=2.4300385410805355e-07}, {"X"=5.36, "Y"=2.3033328004392066e-07}, {"X"=5.37, "Y"=2.1830153687797888e-07}, {"X"=5.38, "Y"=2.0687759787196552e-07}, {"X"=5.39, "Y"=1.9603188091675758e-07}, {"X"=5.4, "Y"=1.8573618445552897e-07}, {"X"=5.41, "Y"=1.7596362609104592e-07}, {"X"=5.42, "Y"=1.6668858377222828e-07}, {"X"=5.43, "Y"=1.5788663945889064e-07}, {"X"=5.44, "Y"=1.495345251671592e-07}, {"X"=5.45, "Y"=1.4161007130161178e-07}, {"X"=5.46, "Y"=1.3409215718354753e-07}, {"X"=5.47, "Y"=1.2696066368812932e-07}, {"X"=5.48, "Y"=1.201964279062823e-07}, {"X"=5.49, "Y"=1.1378119975034591e-07}, {"X"=5.5, "Y"=1.0769760042543276e-07}, {"X"=5.51, "Y"=1.0192908269135293e-07}, {"X"=5.52, "Y"=9.645989284273384e-08}, {"X"=5.53, "Y"=9.127503433766477e-08}, {"X"=5.54, "Y"=8.636023300780988e-08}, {"X"=5.55, "Y"=8.17019037854322e-08}, {"X"=5.56, "Y"=7.728711888522921e-08}, {"X"=5.57, "Y"=7.310357738120935e-08}, {"X"=5.58, "Y"=6.913957612112398e-08}, {"X"=5.59, "Y"=6.538398192315145e-08}, {"X"=5.6, "Y"=6.182620500165857e-08}, {"X"=5.61, "Y"=5.84561735709005e-08}, {"X"=5.62, "Y"=5.526430957749716e-08}, {"X"=5.63, "Y"=5.2241505514424374e-08}, {"X"=5.64, "Y"=4.937910227110449e-08}, {"X"=5.65, "Y"=4.666886797594257e-08}, {"X"=5.66, "Y"=4.410297778937308e-08}, {"X"=5.67, "Y"=4.167399460712351e-08}, {"X"=5.68, "Y"=3.9374850634998504e-08}, {"X"=5.69, "Y"=3.7198829798016034e-08}, {"X"=5.7, "Y"=3.513955094820434e-08}, {"X"=5.71, "Y"=3.319095183679538e-08}, {"X"=5.72, "Y"=3.134727381791979e-08}, {"X"=5.73, "Y"=2.960304725223005e-08}, {"X"=5.74, "Y"=2.795307758015465e-08}, {"X"=5.75, "Y"=2.6392432035705735e-08}, {"X"=5.76, "Y"=2.4916426972950992e-08}, {"X"=5.77, "Y"=2.352061577839084e-08}, {"X"=5.78, "Y"=2.2200777343579013e-08}, {"X"=5.79, "Y"=2.0952905073377047e-08}, {"X"=5.8, "Y"=1.9773196406244675e-08}, {"X"=5.81, "Y"=1.865804282394618e-08}, {"X"=5.82, "Y"=1.7604020328985783e-08}, {"X"=5.83, "Y"=1.6607880368992047e-08}, {"X"=5.84, "Y"=1.5666541188132572e-08}, {"X"=5.85, "Y"=1.4777079586480055e-08}, {"X"=5.86, "Y"=1.3936723069047392e-08}, {"X"=5.87, "Y"=1.3142842366982143e-08}, {"X"=5.88, "Y"=1.239294431415013e-08}, {"X"=5.89, "Y"=1.168466506304987e-08}, {"X"=5.9, "Y"=1.1015763624682308e-08}, {"X"=5.91, "Y"=1.0384115717656327e-08}, {"X"=5.92, "Y"=9.78770791244118e-09}, {"X"=5.93, "Y"=9.22463205728272e-09}, {"X"=5.94, "Y"=8.693079972880173e-09}, {"X"=5.95, "Y"=8.191338403479174e-09}, {"X"=5.96, "Y"=7.717784212570529e-09}, {"X"=5.97, "Y"=7.270879811900108e-09}, {"X"=5.98, "Y"=6.8491688129857586e-09}, {"X"=5.99, "Y"=6.451271890811751e-09}, {"X"=6.0, "Y"=6.075882849823286e-09}, {"X"=6.01, "Y"=5.7217648827798965e-09}, {"X"=6.02, "Y"=5.38774701344276e-09}, {"X"=6.03, "Y"=5.072720714470481e-09}, {"X"=6.04, "Y"=4.775636692282276e-09}, {"X"=6.05, "Y"=4.4955018310132455e-09}, {"X"=6.06, "Y"=4.231376288039894e-09}, {"X"=6.07, "Y"=3.982370733890178e-09}, {"X"=6.08, "Y"=3.747643729676039e-09}, {"X"=6.09, "Y"=3.526399235495381e-09}] ("Normal Distribution")
    }
    frame #1 {
      w5 = 16  # ch
      # "표준 정규 분표표 XY값 입력"
      n3 = for {
        N: w5 -> [_]
        tunnel: [w9] -> w7 mode=indexing
        i -> [w15]
        # "커서 생성"
        n4 = Increment(x=w15) -> (x+1=w8:i32)
        n5 = call-poly <vilib>:"Random Number (Range).vi"("lower bound (0)"=u64 255, "upper bound (100)"=u64 16711680) -> ("number"=w16:u64)  [unwired: 9 in]
        n6 = Format Into String(format string="%dch" ("포맷 문자열"), w8) -> (resulting string=w13:string)  [unwired: 2 in, 1 out]
        n7 = To Unsigned Long Integer(number=w16) -> (unsigned 32bit integer=w10:u32)
        n8 = Bundle By Name(cluster=T1 {"Name"="CH1", "Color"=16715776, "Style"=4, "Point Style"=2, "Name Visible"=TRUE, "Allow Drag"=FALSE, "Cursor Mode"=1, "Plot"=-1, "Index"=669, "Position"={"X"=0.59, "Y"=0.33521319948710615}, "X Scale"=0, "Y Scale"=0, "Watch Plots"=[], "Watch All Plots"=FALSE, "Plot Area"=0, "Label Offset"={"X"=-0.0013207547169812317, "Y"=0.014565887405382782}}, "Name"=w13, "Color"=w10) -> (w9:T1)
      }
      n9 = property on="xyGraph" class="XYGraph (엄격한)"("CrsrList"=w7) -> (error out=w6:errorcluster)  [unwired: 2 in, 1 out]
    }
  }
  n10 = while {
    tunnel: w2 -> [_]
    tunnel: w1 -> [w19]
    stop <- "stop" stop-if-true
    # "표준 편차 계산"
    # "평균 계산"
    # "sigma Loop"
    n11 = for {
      N: w19 -> [_]
      tunnel: [w33] -> w18 mode=indexing
      # "값 임의 입력"
      n12 = call-poly <vilib>:"Random Number (Range).vi"("lower bound (0)"=-100.0, "upper bound (100)"=100.0) -> ("number"=w33:dbl)  [unwired: 9 in]
    }
    n13 = call <vilib>:"Measures of Mean.vi"("percent (trim)"=25.0, "type"=T2."trimmed", "x array"=w18) -> ("mean value"=w23:dbl)  [unwired: 7 in, 1 out]
    n14 = for {
      tunnel: w18 -> [w41] mode=indexing
      tunnel: [w40] -> w29 mode=indexing
      tunnel: w23 -> [w39]
      # "편차"
      n15 = Subtract(x=w41, y=w39) -> (x-y=w40:dbl)
    }
    n16 = Square(x=w29) -> (x^2=w27:dbl[])
    n17 = Array Size(array=w29) -> (size(s)=w24:i32)
    n18 = Add Array Elements(numeric array=w27) -> (sum=w25:dbl)
    n19 = Decrement(x=w24) -> (x-1=w26:i32)
    n20 = Divide(x=w25, y=w26) -> (x/y=w28:dbl)
    n21 = Square Root(x=w28) -> (sqrt(x)=w30:dbl)
    n22 = for {
      tunnel: w30 -> [w38]
      tunnel: w29 -> [w37] mode=indexing
      tunnel: [w36] -> w20 mode=indexing
      # "편차/표준편차 = 표준정규분포"
      n23 = Divide(x=w37, y=w38) -> (x/y=w36:dbl)
    }
    n24 = for {
      N: w19 -> [_]
      tunnel: w20 -> [w42] mode=indexing
      i -> [w43]
      n25 = property on="xyGraph" class="XYGraph (엄격한)"("Active Cursor"=w43, "Cursor.Cursor X"=w42) -> ()  [unwired: 2 in, 2 out]
    }
    n26 = Wait Until Next ms Multiple(millisecond multiple=u32 1000 ("ms 배수")) -> ()  [unwired: 1 out]
  }
